vi "Graphical User Interface - Frigg.vi"() -> ()   [LabVIEW 2014]
uses:
  <vilib>/robotics/Controls/Attitude Indicator/Attitude Indicator.xctl
  <vilib>/robotics/Controls/Compass Indicator/Compass Indicator.xctl
  <vilib>/Platform/TimedLoop/XDataNode/timing_clust.ctl
  <vilib>/Platform/TimedLoop/XDataNode/nitl_modes.ctl
  <vilib>/Platform/TimedLoop/XDataNode/wakeup.ctl
  <vilib>/imath/engines/lvmath2/RunTimeEngine/Managers/WorkSpace/UID Generator.vi
  <vilib>/imath/engines/lvmath2/RunTimeEngine/IndexRead/NIMS V(S).vi
  <instcachedir>/0/NIMS V(S)_0488751826AF41519A22953C041130DC.lvgen/NIMS V(S)_0488751826AF41519A22953C041130DC_000.vi
  <vilib>/imath/engines/lvmath2/RunTimeEngine/RunTimeType/NIMS_RunTimeType_From StrictType (excl LVString).vi
  <instcachedir>/0/NIMS_RunTimeType_From StrictType (excl LVString)_15A5391EEA9C4AACB9955AC755B83D29.lvgen/NIMS_RunTimeType_From StrictType (excl LVString)_15A5391EEA9C4AACB9955AC755B83D29_000.vi
  <vilib>/imath/engines/lvmath2/RunTimeEngine/ErrorHandling/NIMS_Create Error From Enums.vi
  <vilib>/imath/engines/lvmath2/RunTimeEngine/LocalVariableDefStatement/MC_LocalVariableDefStatement_Display.vi
  <vilib>/imath/engines/lvmath2/RunTimeEngine/Managers/SymbolTable/Clear UID.vi
  <vilib>/imath/engines/lvmath2/RunTimeEngine/NodeEndStatement/NIMS_NodeEndStatement_Output.vi
  <instcachedir>/0/NIMS_NodeEndStatement_Output_53EC0D466D134D7ABD903AC30B43404B.lvgen/NIMS_NodeEndStatement_Output_53EC0D466D134D7ABD903AC30B43404B_010.vi
  <instcachedir>/0/NIMS_NodeEndStatement_Output_53EC0D466D134D7ABD903AC30B43404B.lvgen/NIMS_NodeEndStatement_Output_53EC0D466D134D7ABD903AC30B43404B_012.vi
  <vilib>/imath/engines/lvmath2/RunTimeEngine/ErrorHandling/NIMS_Finalize Error.vi
  <vilib>/Platform/TimedLoop/XDataNode/XDataNode.xnode
  <vilib>/Platform/TimedLoop/XDataNode/XDNodeRunTimeDep.lvlib
  <vilib>/imath/engines/lvmath2/RunTimeEngine/Managers/SymbolTable/NIMS_WorkSpace.lvlib
panel:
  out "INTERFACE RUNNING":bool
  out "!":bool
  out "Des Head. [deg] 2":dbl format="%#.1f"
  in  "Start New LogFile":bool
  out "Altitide [m]":dbl format="%#.2f"
  out "Des. Altitude":dbl format="%#.2f"
  out "Head. [deg]":dbl format="%#.1f"
  out "Des Head. [deg]":dbl format="%#.1f"
  out "Depth [m]":dbl format="%#.2f"
  out "Des Depth [m]":dbl format="%#.2f"
  out "ALTITUDE":cluster{dbl, dbl}(slide) scale=0.0..10.0
  out "DEPTH":cluster{dbl, dbl}(slide)
  out "DESIRED (red) / ESTIMATED (blue) HEADING":cluster{dbl, dbl}(slide) scale=0.0..360.0
  out "Compass Indicator":dbl(xcontrol)
  out "Attitude Indicator":cluster{"Roll":dbl, "Pitch":dbl}(xcontrol)
  out "POSITION":bool
  in  "Set altitude":bool
  in  "Altitude Button":bool
  in  "Reset Signal \nProcessing":bool
  in  "COLLECTION\nUNIT":bool
  out "Between Setpoints":bool
  out "Auto Par. on Reference Model":bool
  out "MapViewAct":bool
  in  "Reset ROV":bool
  in  "Reset Controller":bool
  in  "Reset Observer":bool
  out "DEPTH":bool
  out "HEADING":bool
  in  "Reset Plots":bool
  in  "Start Button":bool
  out "Using Observer":bool
  in  "SetOrigin":bool
  out "AdvViewAct":bool
  out "ALTITUDE BEAMS":bool[](array[boolean])
  out "Help Field":string
  in  "Vessel Data":bool
  in  "CAMERAS":bool
  in  "MANIPULATOR":bool
  in  "LIGHTS":bool
  out "Status Messages":string[][](table)
  in  "Connect Button":bool
  in  "DP Button":bool
  in  "Stop Button":bool
  in  "Joystick Button":bool
  in  "Tracking Button":bool
  out "SONAR ALT":bool
  out "YAW RATE":bool
  out "SWAY":bool
  out "SURGE":bool
  out "HEADING":bool
  out "DEPTH":bool
  out "EAST":bool
  out "NORTH":bool
  in  "WindowsMediaPlayer":refnum<k7>(container)
  # "AUR-Lab Underwater Operations Control"
  # "ROV info"
  # "SENSORS STATE"
  # "N"
  # "E"
  # "S"
  # "W"
  # "N"
  # "MISSION CONTROL"
  # "DISTANCE ROV-SHIP\non x-y plane"
  # "AUTOPILOT FUNCTIONS"
  # "CONTROL PANEL"
  # "RESET PANEL"
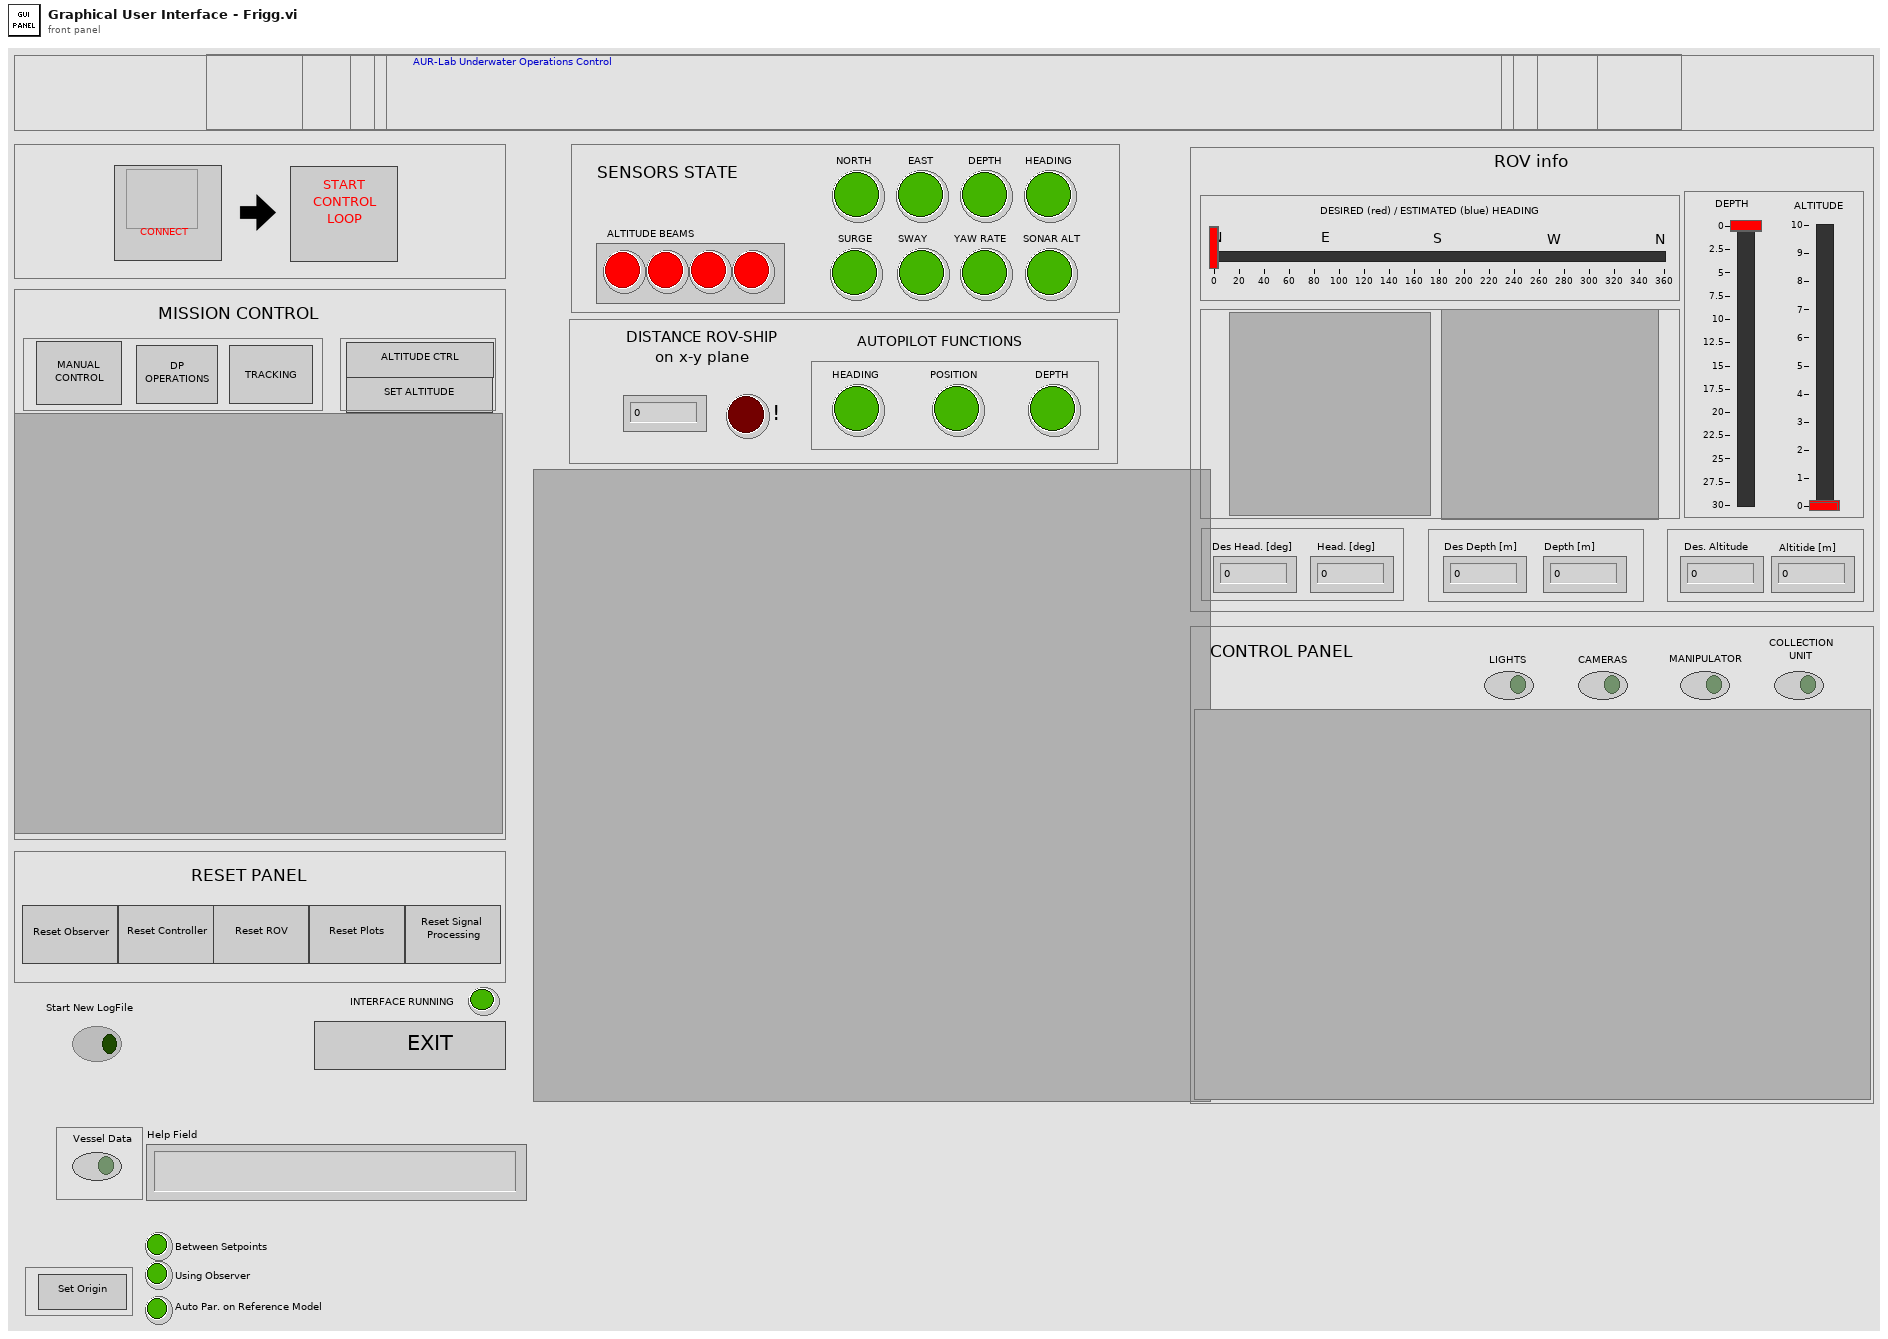
[diagram p1: front panel]
types:
  T1 = enum16{"open", "replace", "create", "open or create", "replace or create", "replace or create with confirmation"}
  T2 = typedef "XDNodeRunTimeDep.lvlib/timing_clust.ctl" = cluster{"Expected End [f-1]":u64, "Actual End [f-1]":u64, "Finished Late? [f-1]":bool, "Expected End [i-1]":u64, "Actual End [i-1]":u64, "Finished Late? [i-1]":bool, "Expected Start [i]":u64, "Actual Start [i]":u64, "Expected Start [f]":u64, "Actual Start [f]":u64, "Source Name":string, "Structure Name":string, "Period":i64, "Deadline":i64, "Offset":i64, "Start":i64, "Priority":i32, "Timeout":i32, "Mode":T3, "Wakeup Reason":T4, "Error":errorcluster, "Source Type":string, "Secondary Source Type":string, "Global End Time":u64, "Global Start Time":u64, "Frame Duration":u64, "Iteration Duration":u64, "Assigned CPU":i32, "I/O Scan Engine Mode":u32}
  T3 = typedef "XDNodeRunTimeDep.lvlib/nitl_modes.ctl" = enum32{"No Change", "Process missed periods, maintain original phase", "Discard missed periods, maintain original phase", "Process missed periods, ignore original phase", "Discard missed periods, ignore original phase"}
  T4 = typedef "XDNodeRunTimeDep.lvlib/wakeup.ctl" = enum32{"Normal", "Aborted", "Asynchronous wakeup", "Timing source error", "Timed loop error", "Timeout"}
  T5 = enum8{"Enabled", "Disabled", "Disabled and Grayed Out"}
  T6 = cluster{"Des Heading [deg]":dbl, "Heading [deg]":dbl}
  T7 = cluster{"Altitude Desired":dbl, "Altitide Estimated":dbl}
  T8 = cluster{"Des Heading [deg]":dbl, "Des Heading [deg]":dbl}
  T9 = cluster{"Shift":bool, "Ctrl":bool, "Alt":bool, "Cmd":bool, "Opt":bool}
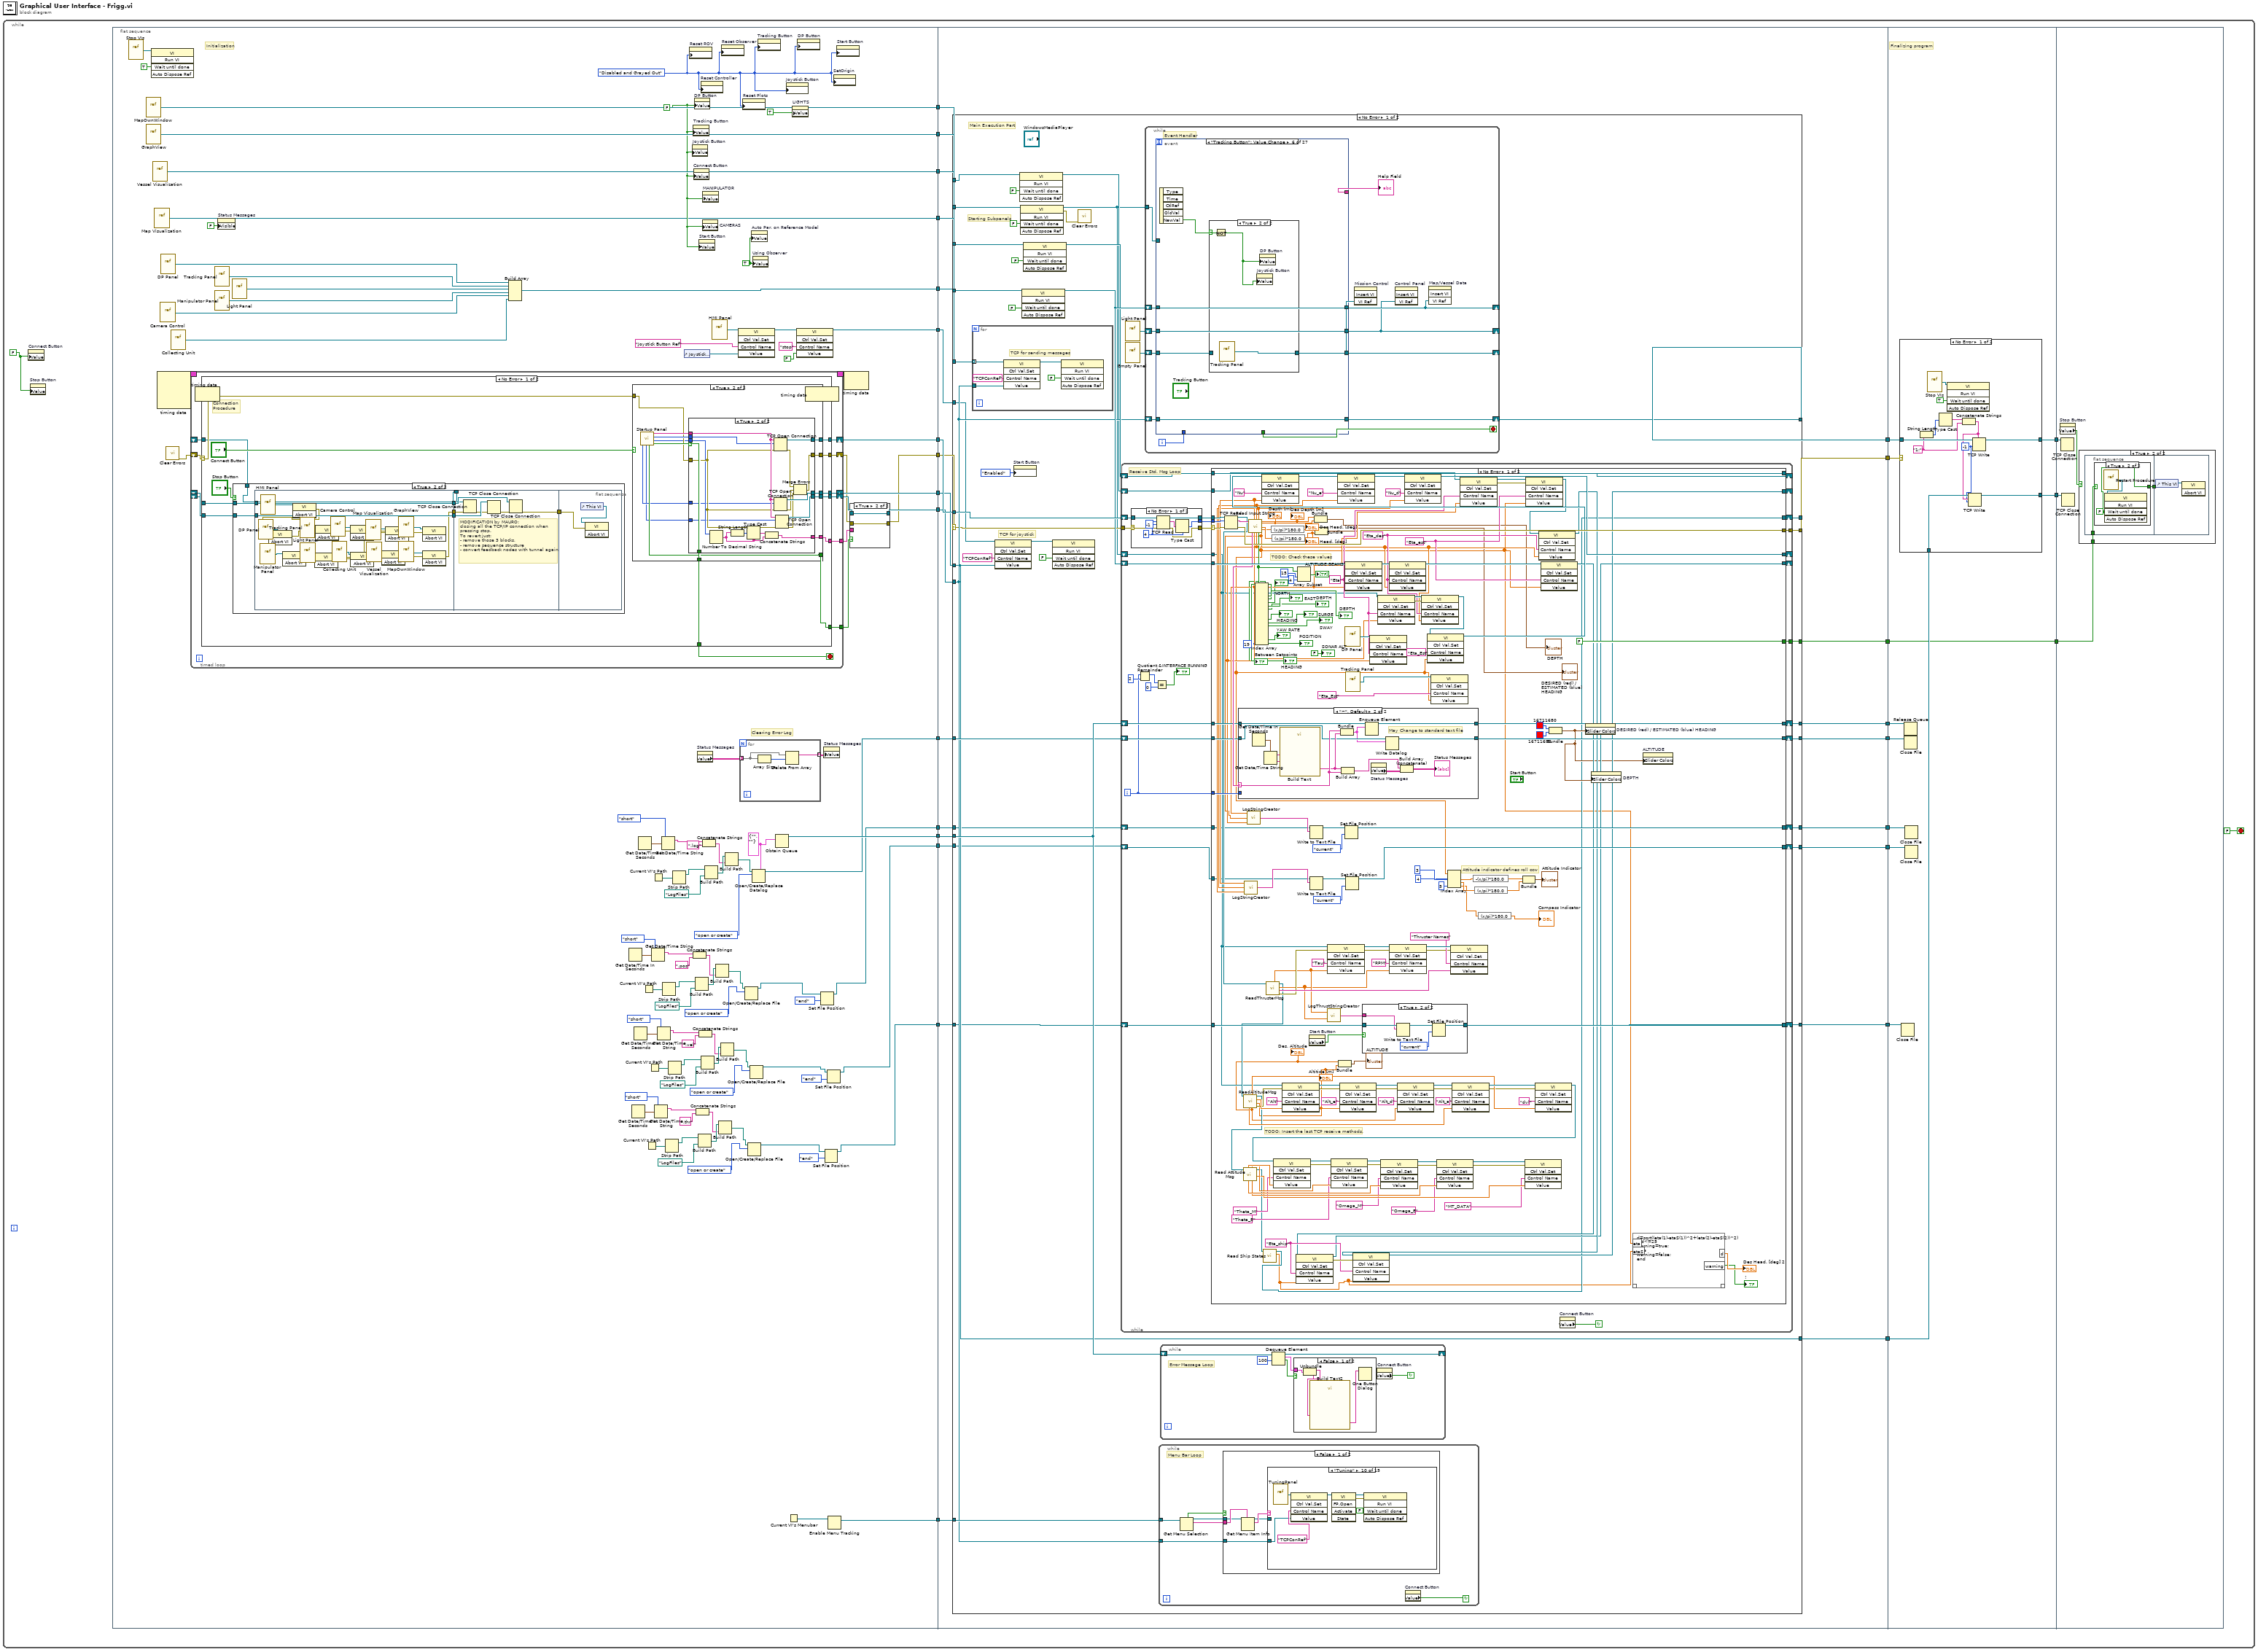
[diagram p0: block diagram]
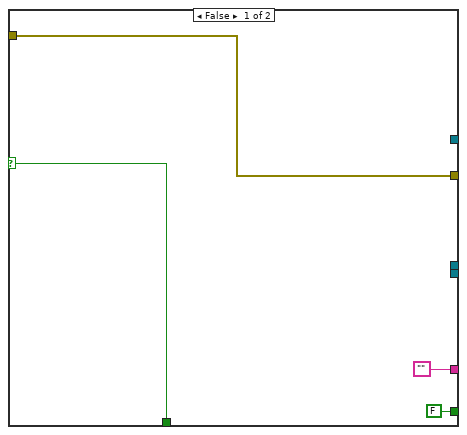
[diagram p3: hidden frame]
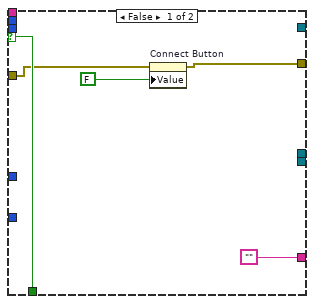
[diagram p4: hidden frame]
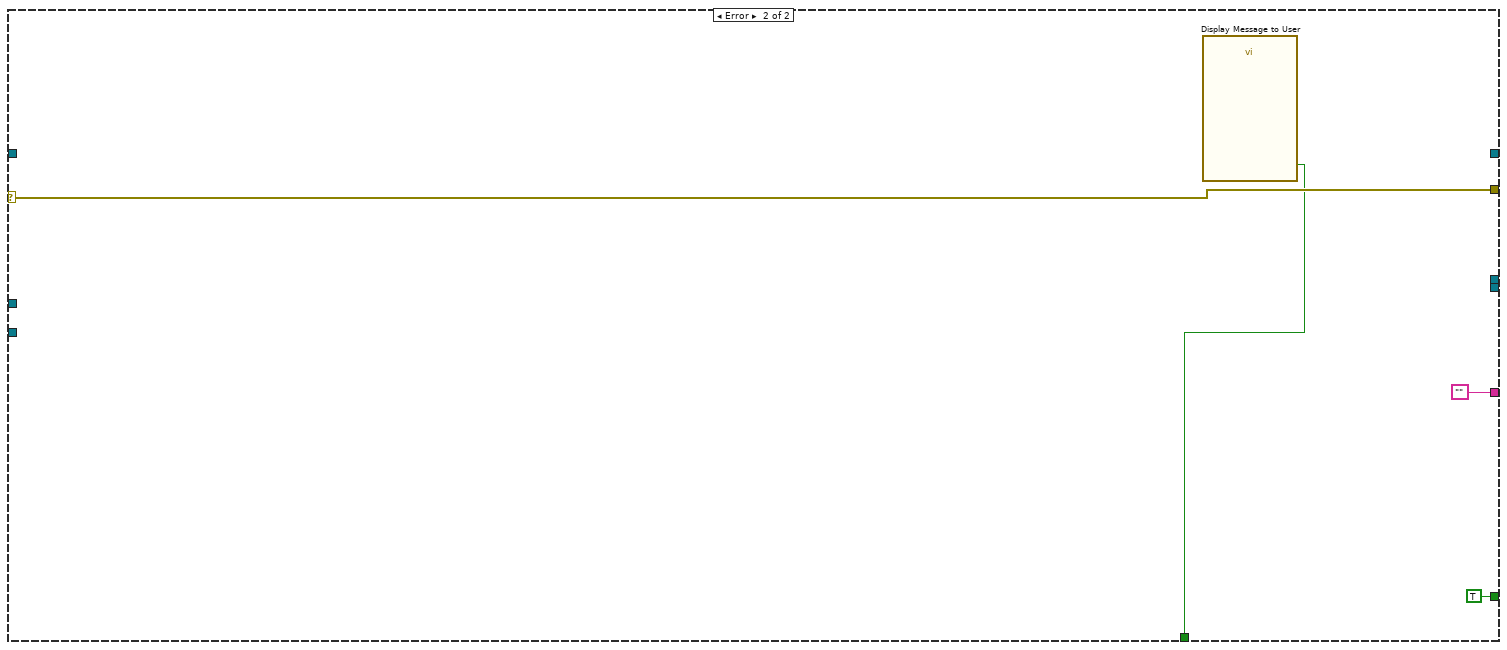
[diagram p5: hidden frame]
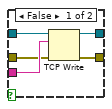
[diagram p6: hidden frame]
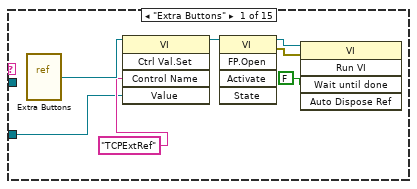
[diagram p7: hidden frame]
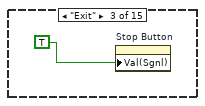
[diagram p9: hidden frame]
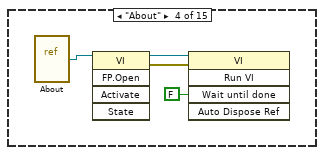
[diagram p10: hidden frame]
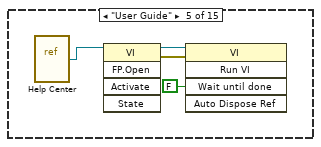
[diagram p11: hidden frame]
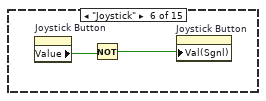
[diagram p12: hidden frame]
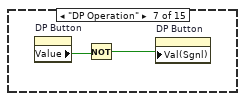
[diagram p13: hidden frame]
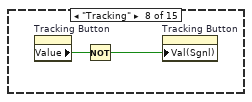
[diagram p14: hidden frame]
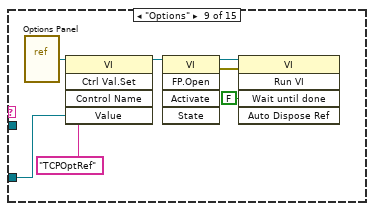
[diagram p15: hidden frame]
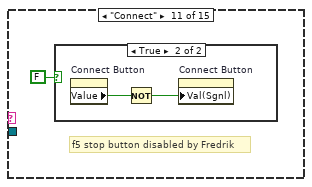
[diagram p16: hidden frame]
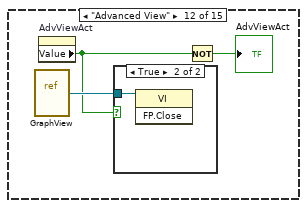
[diagram p18: hidden frame]
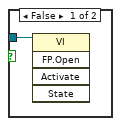
[diagram p19: hidden frame]
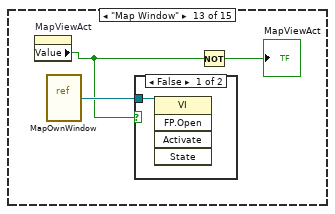
[diagram p20: hidden frame]
diagram:
  n1 = while {
    stop <- FALSE stop-if-true
    w2 = FALSE
    n2 = property on="Connect Button" class="Bool (strict)"("Value"=w2) -> ()  [unwired: 2 in, 2 out]
    n3 = property on="Stop Button" class="Bool (strict)"("Value"=w2) -> ()  [unwired: 2 in, 2 out]
    n4 = flat-sequence {
      tunnel: [w126] -> w30
      tunnel: [w31] -> w29
      tunnel: [w123] -> w28
      tunnel: [w117] -> w27
      tunnel: [w32] -> w26
      tunnel: [w113] -> w25
      tunnel: [w109] -> w23
      tunnel: [w107] -> w19
      tunnel: [w51] -> w18
      tunnel: [w54] -> w14
      tunnel: [w104] -> w13
      tunnel: [w91] -> w12
      tunnel: [w40] -> w8
      tunnel: [w38] -> w6
      tunnel: [w36] -> w5
      tunnel: [w57] -> w3
      tunnel: w30 -> [w271]
      tunnel: [w251] -> w22
      tunnel: w29 -> [w274]
      tunnel: w28 -> [w273]
      tunnel: w27 -> [w272]
      tunnel: w26 -> [w270]
      tunnel: w25 -> [w269]
      tunnel: [w264] -> w21
      tunnel: w23 -> [w268]
      tunnel: [w267] -> w20
      tunnel: w19 -> [w266]
      tunnel: w18 -> [w265]
      tunnel: [w263] -> w17
      tunnel: [w262] -> w15
      tunnel: w14 -> [w261]
      tunnel: w13 -> [w260]
      tunnel: w12 -> [w259]
      tunnel: [w258] -> w11
      tunnel: w8 -> [w257]
      tunnel: [w256] -> w7
      tunnel: w6 -> [w254]
      tunnel: w5 -> [w255]
      tunnel: [w253] -> w4
      tunnel: w3 -> [w252]
      tunnel: [w250] -> w1
      tunnel: w22 -> [w1109]
      tunnel: w21 -> [w1108]
      tunnel: w20 -> [w1107]
      tunnel: w17 -> [w1106]
      tunnel: [w1105] -> w16
      tunnel: w15 -> [w1105]
      tunnel: w11 -> [w1104]
      tunnel: [w1103] -> w10
      tunnel: [w1102] -> w9
      tunnel: w7 -> [w1101]
      tunnel: w4 -> [w1100]
      tunnel: w1 -> [w1099]
      tunnel: w16 -> [w1128]
      tunnel: w10 -> [w1127]
      tunnel: w9 -> [w1126]
      frame #0 {
        w50 = T5."Disabled and Grayed Out" ("Disabled")
        w56 = TRUE ("Using Observer")
        w92 = cluster{string, string} {"", ""}
        w43 = FALSE
        # "Clearing Error Log"
        # "Initialization"
        n5 = vi-ref "Stop VIs.vi"() -> (w48:refnum<vi>)
        n6 = vi-ref "MapOwnWindow.vi"() -> (w57:refnum<vi>)
        n7 = vi-ref "GraphView.vi"() -> (w104:refnum<vi>)
        n8 = invoke class="VI" method="Run VI"(reference=w48, "Wait until done"=TRUE ("Wait Until Done")) -> ()  [unwired: 3 in, 5 out]
        n9 = vi-ref "Vessel Visualization.vi"() -> (w123:refnum<vi>)
        n10 = vi-ref "Map Visualization.vi"() -> (w31:refnum<vi>)
        n11 = node-c288() -> (w46:T2)  [unwired: 4 in]
        n12 = vi-ref "Camera Control.vi"() -> (w118:refnum<vi>)
        n13 = vi-ref "DP Panel.vi"() -> (w122:refnum<vi>)
        n14 = call <vilib>:"Clear Errors.vi"() -> ("error out"=w105:errorcluster)  [unwired: 6 in, 1 out]
        n15 = vi-ref "Collecting Unit.vi"() -> (w44:refnum<vi>)
        n16 = timed-loop {
          shift-right: [w134] -> w52
          shift-left: w105 -> [w133]
          tunnel: [w131] -> w55
          tunnel: [w130] -> w47
          timing: w46 -> [_]
          timing-out: [_] -> w45
          shift-right: [w137] -> w126
          shift-left: _ -> [w129]
          shift-right: [w136] -> w113
          shift-left: _ -> [w128]
          shift-right: [w132] -> w53
          shift-left: _ -> [w127]
          stop <- w135 stop-if-true
          n17 = node-c288() -> ()  [unwired: 1 in, 1 out]
          n18 = case shown="No Error" w133 {
            selector: w133 -> [w147 w237]
            tunnel: [w152 _] -> w137
            tunnel: [w151 _] -> w136
            tunnel: [w150 w236] -> w135
            tunnel: [w148 w237] -> w134
            tunnel: [w146 _] -> w132
            tunnel: [w145 ""] -> w131
            tunnel: [w143 TRUE ("Restart Out")] -> w130
            tunnel: w129 -> [w140 _]
            tunnel: w128 -> [w142 _]
            tunnel: w127 -> [w141 _]
            frame No Error {
              # "Connection\nProcedure"
              n19 = case shown="True" "Stop Button" {
                tunnel: w142 -> [_ w159]
                tunnel: w141 -> [_ w158]
                tunnel: w140 -> [_ w155]
                frame False {
                }
                frame True {
                  n20 = flat-sequence {
                    tunnel: w158 -> [w182]
                    tunnel: w159 -> [w183]
                    tunnel: [w183] -> w157
                    tunnel: [w182] -> w156
                    tunnel: [w160] -> w154
                    tunnel: w157 -> [w190]
                    tunnel: w156 -> [w189]
                    tunnel: w155 -> [w188]
                    tunnel: w154 -> [w187]
                    tunnel: [w184] -> w153
                    tunnel: w153 -> [w191]
                    frame #0 {
                      n21 = vi-ref "DP Panel.vi"() -> (w181:refnum<vi>)
                      n22 = vi-ref "Manipulator Panel.vi"() -> (w176:refnum<vi>)
                      n23 = vi-ref "HMI Panel.vi"() -> (w162:refnum<vi>)
                      n24 = invoke class="VI" method="Abort VI"(reference=w162) -> (error out=w161:errorcluster)  [unwired: 2 in, 2 out]
                      n25 = invoke class="VI" method="Abort VI"(reference=w181, error in=w161) -> (error out=w171:errorcluster)  [unwired: 1 in, 2 out]
                      n26 = vi-ref "Tracking Panel.vi"() -> (w180:refnum<vi>)
                      n27 = vi-ref "Light Panel.vi"() -> (w175:refnum<vi>)
                      n28 = invoke class="VI" method="Abort VI"(reference=w180, error in=w171) -> (error out=w170:errorcluster)  [unwired: 1 in, 2 out]
                      n29 = vi-ref "Camera Control.vi"() -> (w179:refnum<vi>)
                      n30 = vi-ref "Collecting Unit.vi"() -> (w174:refnum<vi>)
                      n31 = invoke class="VI" method="Abort VI"(reference=w179, error in=w170) -> (error out=w169:errorcluster)  [unwired: 1 in, 2 out]
                      n32 = vi-ref "Map Visualization.vi"() -> (w178:refnum<vi>)
                      n33 = vi-ref "Vessel Visualization.vi"() -> (w173:refnum<vi>)
                      n34 = invoke class="VI" method="Abort VI"(reference=w178, error in=w169) -> (error out=w168:errorcluster)  [unwired: 1 in, 2 out]
                      n35 = vi-ref "GraphView.vi"() -> (w177:refnum<vi>)
                      n36 = vi-ref "MapOwnWindow.vi"() -> (w172:refnum<vi>)
                      n37 = invoke class="VI" method="Abort VI"(reference=w177, error in=w168) -> (error out=w167:errorcluster)  [unwired: 1 in, 2 out]
                      n38 = invoke class="VI" method="Abort VI"(reference=w176, error in=w167) -> (error out=w166:errorcluster)  [unwired: 1 in, 2 out]
                      n39 = invoke class="VI" method="Abort VI"(reference=w175, error in=w166) -> (error out=w165:errorcluster)  [unwired: 1 in, 2 out]
                      n40 = invoke class="VI" method="Abort VI"(reference=w174, error in=w165) -> (error out=w164:errorcluster)  [unwired: 1 in, 2 out]
                      n41 = invoke class="VI" method="Abort VI"(reference=w173, error in=w164) -> (error out=w163:errorcluster)  [unwired: 1 in, 2 out]
                      n42 = invoke class="VI" method="Abort VI"(reference=w172, error in=w163) -> (error out=w160:errorcluster)  [unwired: 1 in, 2 out]
                    }
                    frame #1 {
                      # "MODIFICATION by MAURO:\nclosing all the TCP/IP connection when\npressing stop.\nTo revert just:\n- remove those 3 blocks, \n- remove sequence structure\n- convert feedback nodes with tunnel again"
                      n43 = TCP Close Connection(connection ID=w188, error in (no error)=w187) -> (error out=w186:errorcluster)  [unwired: 1 in, 1 out]
                      n44 = TCP Close Connection(connection ID=w190, error in (no error)=w186) -> (error out=w185:errorcluster)  [unwired: 1 in, 1 out]
                      n45 = TCP Close Connection(connection ID=w189, error in (no error)=w185) -> (error out=w184:errorcluster)  [unwired: 1 in, 1 out]
                    }
                    frame #2 {
                      n46 = control-ref of="This VI"() -> (w192:refnum<vi>)
                      n47 = invoke class="VI" method="Abort VI"(reference=w192, error in=w191) -> ()  [unwired: 1 in, 3 out]
                    }
                  }
                }
              }
              n48 = case shown="True" "Connect Button" {
                selector: "Connect Button" -> [w196 _]
                tunnel: [_ w210] -> w152
                tunnel: [_ w209] -> w151
                tunnel: [w196 w208] -> w150
                tunnel: [w195 w207] -> w148
                tunnel: w147 -> [w195 w202]
                tunnel: [_ w206] -> w146
                tunnel: ["" w200] -> w145
                tunnel: [FALSE ("Restart Out") w199] -> w143
                frame False {
                }
                frame True {
                  n49 = call "Startup Panel.vi"() -> ("Bool Out"=w204:bool, "ROV Selector Out"=w201:u16, "Port Number Recv Out 1"=w203:u16, "IP Address Out"=w205:string, "Restart Out"=w199:bool, "Port Number  Send Out"=w197:u16, "Port Number Joyst. Out"=w198:u16)  [unwired: 5 in]
                  n50 = case shown="True" w204 {
                    selector: w204 -> [w214 w230]
                    tunnel: [_ w233] -> w210
                    tunnel: [_ w232] -> w209
                    tunnel: w205 -> [_ w231]
                    tunnel: w203 -> [_ w224]
                    tunnel: [w214 w230] -> w208
                    tunnel: w202 -> [w213 w228]
                    tunnel: [w212 w225] -> w207
                    tunnel: [_ w229] -> w206
                    tunnel: w201 -> [_ w223]
                    tunnel: ["" w219] -> w200
                    tunnel: w198 -> [_ w218]
                    tunnel: w197 -> [_ w217]
                    frame False {
                      n51 = property on="Connect Button" class="Bool (strict)"(error in=w213, "Value"=FALSE ("Connect Button")) -> (error out=w212:errorcluster)  [unwired: 1 in, 1 out]
                    }
                    frame True {
                      n52 = Number To Decimal String(number=w223) -> (decimal integer string=w220:string)  [unwired: 1 in]
                      n53 = String Length(string=w220) -> (length=w222:i32)
                      n54 = Type Cast(type=w220, x=w222) -> (*(type *) &x=w221:string)
                      n55 = Concatenate Strings(w221, w220) -> (w219:string)
                      n56 = TCP Open Connection(address=w231, remote port or service name=w224, error in (no error)=w228) -> (connection ID=w233:refnum<k5>, error out=w216:errorcluster)  [unwired: 2 in]
                      n57 = TCP Open Connection(address=w231, remote port or service name=w218, error in (no error)=w228) -> (connection ID=w232:refnum<k5>, error out=w227:errorcluster)  [unwired: 2 in]
                      n58 = TCP Open Connection(address=w231, remote port or service name=w217, error in (no error)=w228) -> (connection ID=w229:refnum<k5>, error out=w226:errorcluster)  [unwired: 2 in]
                      n59 = Merge Errors(w216, w227, w226) -> (w225:errorcluster)
                    }
                  }
                }
              }
            }
            frame Error {
              n60 = call "Display Message to User"() -> ("OK"=w236:bool)  [unwired: 10 in, 1 out]
            }
          }
          n61 = node-c288() -> ()  [unwired: 1 in, 1 out]
        }
        n62 = vi-ref "Tracking Panel.vi"() -> (w121:refnum<vi>)
        n63 = vi-ref "Manipulator Panel.vi"() -> (w119:refnum<vi>)
        n64 = property on="Status Messages" class="Tbl (strict)"("Visible"=FALSE) -> ()  [unwired: 2 in, 2 out]
        n65 = vi-ref "Light Panel.vi"() -> (w120:refnum<vi>)
        n66 = Build Array(w122, w121, w120, w119, w118, w44) -> (w117:refnum<vi>[])
        n67 = Get Date/Time In Seconds() -> (seconds since 1Jan1904=w87:timestamp)
        n68 = Get Date/Time In Seconds() -> (seconds since 1Jan1904=w65:timestamp)
        n69 = Get Date/Time In Seconds() -> (seconds since 1Jan1904=w76:timestamp)
        n70 = Get Date/Time In Seconds() -> (seconds since 1Jan1904=w100:timestamp)
        n71 = Current VI's Path() -> (path=w90:path)
        n72 = Current VI's Path() -> (path=w68:path)
        n73 = Current VI's Path() -> (path=w79:path)
        n74 = Get Date/Time String(date format (0)=enum16{"short", "long", "abbreviated"}."short", seconds (now)=w87) -> (date string=w86:string)  [unwired: 1 in, 1 out]
        n75 = Current VI's Path() -> (path=w103:path)
        n76 = Get Date/Time String(date format (0)=enum16{"short", "long", "abbreviated"}."short", seconds (now)=w65) -> (date string=w64:string)  [unwired: 1 in, 1 out]
        n77 = Get Date/Time String(date format (0)=enum16{"short", "long", "abbreviated"}."short", seconds (now)=w76) -> (date string=w75:string)  [unwired: 1 in, 1 out]
        n78 = Get Date/Time String(date format (0)=enum16{"short", "long", "abbreviated"}."short", seconds (now)=w100) -> (date string=w99:string)  [unwired: 1 in, 1 out]
        n79 = Strip Path(path=w90) -> (stripped path=w89:path)  [unwired: 1 out]
        n80 = Strip Path(path=w68) -> (stripped path=w67:path)  [unwired: 1 out]
        n81 = Strip Path(path=w79) -> (stripped path=w78:path)  [unwired: 1 out]
        n82 = Strip Path(path=w103) -> (stripped path=w102:path)  [unwired: 1 out]
        n83 = control-ref of="Joystick Button"() -> (w115:refnum<vi>)
        n84 = property on="Reset ROV" class="Bool"("DisabledEnum"=w50) -> ()  [unwired: 2 in, 2 out]
        n85 = property on="Joystick Button" class="Bool (strict)"("Value"=w43) -> ()  [unwired: 2 in, 2 out]
        n86 = property on="Tracking Button" class="Bool (strict)"("Value"=w43) -> ()  [unwired: 2 in, 2 out]
        n87 = Concatenate Strings(w86, ".pos" ("string")) -> (w83:string)
        n88 = property on="Connect Button" class="Bool (strict)"("Value"=w43) -> ()  [unwired: 2 in, 2 out]
        n89 = property on="DP Button" class="Bool (strict)"("Value"=w43) -> ()  [unwired: 2 in, 2 out]
        n90 = Build Path(base path=w89, name or relative path=path "LogFiles") -> (appended path=w84:path)
        n91 = Concatenate Strings(w64, ".thr" ("string")) -> (w61:string)
        n92 = property on="Status Messages" class="Tbl (strict)"() -> ("Value"=w125:string[][])  [unwired: 2 in, 2 out]
        n93 = Build Path(base path=w67, name or relative path=path "LogFiles") -> (appended path=w62:path)
        n94 = Concatenate Strings(w75, ".vel" ("string")) -> (w72:string)
        n95 = property on="Start Button" class="Bool (strict)"("Value"=w43) -> ()  [unwired: 2 in, 2 out]
        n96 = property on="Reset Controller" class="Bool"("DisabledEnum"=w50) -> ()  [unwired: 2 in, 2 out]
        n97 = Build Path(base path=w78, name or relative path=path "LogFiles") -> (appended path=w73:path)
        n98 = property on="CAMERAS" class="Bool (strict)"("Value"=w43) -> ()  [unwired: 2 in, 2 out]
        n99 = property on="MANIPULATOR" class="Bool (strict)"("Value"=w43) -> ()  [unwired: 2 in, 2 out]
        n100 = Concatenate Strings(w99, ".log" ("string")) -> (w96:string)
        n101 = Build Path(base path=w102, name or relative path=path "LogFiles") -> (appended path=w97:path)
        n102 = vi-ref "HMI Panel.vi"() -> (w116:refnum<vi>)
        n103 = Build Path(base path=w84, name or relative path=w83) -> (appended path=w81:path)
        n104 = Build Path(base path=w62, name or relative path=w61) -> (appended path=w60:path)
        n105 = Build Path(base path=w73, name or relative path=w72) -> (appended path=w71:path)
        n106 = property on="Reset Observer" class="Bool"("DisabledEnum"=w50) -> ()  [unwired: 2 in, 2 out]
        n107 = Build Path(base path=w97, name or relative path=w96) -> (appended path=w93:path)
        n108 = invoke class="VI" method="Ctrl Val.Set"(reference=w116, "Control Name"="Joystick Button Ref", "Value"=w115) -> (reference out=w110:refnum<vi>)  [unwired: 2 in, 4 out]
        n109 = for {
          tunnel: w125 -> [w248] mode=indexing
          tunnel: [w247] -> w124 mode=indexing
          n110 = Array Size(array=w248) -> (size(s)=w249:i32)
          n111 = Delete From Array(array=w248, length=w249) -> (array with subset deleted=w247:string[])  [unwired: 1 in, 1 out]
        }
        n112 = property on="Reset Plots" class="Bool"("DisabledEnum"=w50) -> ()  [unwired: 2 in, 2 out]
        n113 = Open/Create/Replace File(file path (use dialog)=w81, operation (0:open)=T1."open or create") -> (refnum out=w41:refnum<file>)  [unwired: 4 in, 2 out]
        n114 = Open/Create/Replace File(file path (use dialog)=w60, operation (0:open)=T1."open or create") -> (refnum out=w37:refnum<file>)  [unwired: 4 in, 2 out]
        n115 = Open/Create/Replace File(file path (use dialog)=w71, operation (0:open)=T1."open or create") -> (refnum out=w39:refnum<file>)  [unwired: 4 in, 2 out]
        n116 = property on="Auto Par. on Reference Model" class="Bool (strict)"("Value"=w56) -> ()  [unwired: 2 in, 2 out]
        n117 = Open/Create/Replace Datalog(5:w92, 10:T1."open or create" ("operation (0:open)"), 11:w93) -> (3:w91:refnum<k1>)  [unwired: 3 in, 2 out]
        n118 = property on="Using Observer" class="Bool (strict)"("Value"=w56) -> ()  [unwired: 2 in, 2 out]
        n119 = property on="Tracking Button" class="Bool (strict)"("DisabledEnum"=w50) -> ()  [unwired: 2 in, 2 out]
        n120 = Obtain Queue(element data type=w92) -> (queue out=w109:refnum<queue>)  [unwired: 4 in, 2 out]
        n121 = property on="Joystick Button" class="Bool (strict)"("DisabledEnum"=w50) -> ()  [unwired: 2 in, 2 out]
        n122 = Current VI's Menubar() -> (w108:refnum<k9>)
        n123 = property on="LIGHTS" class="Bool (strict)"("Value"=TRUE) -> ()  [unwired: 2 in, 2 out]
        n124 = invoke class="VI" method="Ctrl Val.Set"(reference=w110, "Control Name"="stop", "Value"=FALSE) -> (reference out=w32:refnum<vi>)  [unwired: 2 in, 4 out]
        n125 = property on="DP Button" class="Bool (strict)"("DisabledEnum"=w50) -> ()  [unwired: 2 in, 2 out]
        n126 = Set File Position(refnum=w41, from (0:start)=enum16{"start", "end", "current"}."end") -> (refnum out=w40:refnum<file>)  [unwired: 2 in, 1 out]
        n127 = property on="Status Messages" class="Tbl (strict)"("Value"=w124) -> ()  [unwired: 2 in, 2 out]
        n128 = Set File Position(refnum=w37, from (0:start)=enum16{"start", "end", "current"}."end") -> (refnum out=w36:refnum<file>)  [unwired: 2 in, 1 out]
        n129 = Set File Position(refnum=w39, from (0:start)=enum16{"start", "end", "current"}."end") -> (refnum out=w38:refnum<file>)  [unwired: 2 in, 1 out]
        n130 = Enable Menu Tracking(4:w108) -> (1:w107:refnum<k9>)  [unwired: 2 in, 1 out]
        n131 = property on="SetOrigin" class="Bool"("DisabledEnum"=w50) -> ()  [unwired: 2 in, 2 out]
        n132 = property on="Start Button" class="Bool (strict)"("DisabledEnum"=w50) -> ()  [unwired: 2 in, 2 out]
        n133 = node-c288(w45) -> ()  [unwired: 1 out]
        n134 = case shown="True" w47 {
          tunnel: w55 -> [w244 _]
          tunnel: [w243 w246] -> w54
          tunnel: w53 -> [w242 w246]
          tunnel: w52 -> [w241 w245]
          tunnel: [w240 w245] -> w51
          frame False {
            n135 = TCP Write(connection ID=w242, data in=w244, error in (no error)=w241) -> (connection ID out=w243:refnum<k5>, error out=w240:errorcluster)  [unwired: 1 in, 1 out]
          }
          frame True {
          }
        }
      }
      frame #1 {
        n136 = case shown="No Error" w265 {
          selector: w265 -> [w290 w1092]
          tunnel: [w314 w1097] -> _
          tunnel: w274 -> [w310 _]
          tunnel: w273 -> [w309 _]
          tunnel: w272 -> [w308 _]
          tunnel: w271 -> [w307 w1097]
          tunnel: w270 -> [w275 _]
          tunnel: w269 -> [w289 w1096]
          tunnel: w268 -> [w300 w1098]
          tunnel: [w299 w1098] -> w267
          tunnel: w266 -> [w298 _]
          tunnel: [w289 w1096] -> w264
          tunnel: [w297 w1092] -> w263
          tunnel: [w296 w1090] -> w262
          tunnel: w261 -> [w291 w1085]
          tunnel: w260 -> [w295 _]
          tunnel: w259 -> [w293 w1089]
          tunnel: [w292 w1089] -> w258
          tunnel: w257 -> [w288 w1088]
          tunnel: [w287 w1088] -> w256
          tunnel: w255 -> [w279 w1086]
          tunnel: w254 -> [w286 w1087]
          tunnel: [w285 w1087] -> w253
          tunnel: w252 -> [w284 _]
          tunnel: [w280 w1085] -> w251
          tunnel: [w278 w1086] -> w250
          frame No Error {
            # "TCP for joystick"
            # "Starting Subpanels"
            # "Main Execution Part"
            n137 = for {
              tunnel: w308 -> [w739] mode=indexing
              tunnel: w291 -> [w738]
              # "TCP for sending messages"
              n138 = invoke class="VI" method="Ctrl Val.Set"(reference=w739, "Control Name"="TCPConRef", "Value"=w738) -> (reference out=w741:refnum<vi>)  [unwired: 2 in, 4 out]
              n139 = invoke class="VI" method="Run VI"(reference=w741, "Wait until done"=FALSE) -> ()  [unwired: 3 in, 5 out]
            }
            n140 = invoke class="VI" method="Ctrl Val.Set"(reference=w275, "Control Name"="TCPConRef", "Value"=w289) -> (reference out=w302:refnum<vi>)  [unwired: 2 in, 4 out]
            n141 = property on="Start Button" class="Bool (strict)"("DisabledEnum"=T5."Enabled" ("Disabled")) -> ()  [unwired: 2 in, 2 out]
            n142 = invoke class="VI" method="Run VI"(reference=w284, "Wait until done"=FALSE ("Wait Until Done")) -> (reference out=w282:refnum<vi>)  [unwired: 3 in, 4 out]
            n143 = invoke class="VI" method="Run VI"(reference=w295, "Wait until done"=FALSE ("Wait Until Done")) -> (reference out=w277:refnum<vi>, error out=w276:errorcluster)  [unwired: 3 in, 3 out]
            n144 = invoke class="VI" method="Run VI"(reference=w310, "Wait until done"=FALSE) -> (reference out=w306:refnum<vi>)  [unwired: 3 in, 4 out]
            n145 = invoke class="VI" method="Run VI"(reference=w309, "Wait until done"=FALSE) -> (reference out=w305:refnum<vi>)  [unwired: 3 in, 4 out]
            n146 = invoke class="VI" method="Run VI"(reference=w302, "Wait until done"=FALSE) -> ()  [unwired: 3 in, 5 out]
            n147 = call <vilib>:"Clear Errors.vi"("error in (no error)"=w276) -> ()  [unwired: 5 in, 2 out]
            n148 = while "Timed Loop" {
              shift-right: [w429] -> w314
              shift-left: w307 -> [w432]
              shift-right: [w428] -> _
              shift-left: w306 -> [w406]
              shift-right: [w426] -> _
              shift-left: w305 -> [w427]
              shift-right: [w424] -> w299
              shift-left: w300 -> [w425]
              tunnel: w290 -> [w423]
              tunnel: [w420] -> w297
              tunnel: [w419] -> w296
              shift-right: [w417] -> _
              shift-left: w277 -> [w418]
              shift-right: [w416] -> w292
              shift-left: w293 -> [w415]
              shift-right: [w413] -> w287
              shift-left: w288 -> [w414]
              shift-right: [w411] -> w285
              shift-left: w286 -> [w412]
              shift-right: [w410] -> _
              shift-left: w282 -> [w407]
              shift-right: [w409] -> w278
              shift-left: w279 -> [w408]
              i -> [w402]
              stop <- w421 continue-if-true
              # "Receive Std. Msg Loop"
              n149 = case shown="No Error" w423 {
                selector: w423 -> [w729 w737]
                tunnel: w432 -> [w734 w736]
                tunnel: [w733 w736] -> w431
                tunnel: [w730 0] -> w430
                tunnel: [w728 w737] -> w422
                frame No Error {
                  w731 = 4
                  n150 = TCP Read(connection ID=w734, bytes to read=w731, error in (no error)=w729, 9:-1 ("timeout ms (25000)")) -> (connection ID out=w733:refnum<k5>, data out=w732:string, error out=w728:errorcluster)  [unwired: 1 in]
                  n151 = Type Cast(type=w731, x=w732) -> (*(type *) &x=w730:i32)
                }
                frame Error {
                }
              }
              n152 = Quotient & Remainder(x=w402, y=2) -> (x-y*floor(x/y)=w401:i32)  [unwired: 1 out]
              n153 = Equal?(x=w401, y=0) -> (x = y?=→"INTERFACE RUNNING":bool)
              n154 = case shown="No Error" w422 {
                selector: w422 -> [w577 w721]
                tunnel: w431 -> [w591 w723]
                tunnel: w430 -> [w590 _]
                tunnel: [w439 w723] -> w429
                tunnel: w406 -> [w589 w725]
                tunnel: [w470 w725] -> w428
                tunnel: w427 -> [w558 w726]
                tunnel: [w558 w726] -> w426
                tunnel: w402 -> [w582 _]
                tunnel: w425 -> [w581 w724]
                tunnel: [w580 w724] -> w424
                tunnel: [w576 w721] -> w420
                tunnel: [FALSE ("Yes") w717] -> w419
                tunnel: w418 -> [w503 w716]
                tunnel: [w559 w716] -> w417
                tunnel: [w566 w715] -> w416
                tunnel: w415 -> [w565 w715]
                tunnel: w414 -> [w478 w714]
                tunnel: [w557 w714] -> w413
                tunnel: w412 -> [w477 w713]
                tunnel: [w552 w713] -> w411
                tunnel: w407 -> [w547 w712]
                tunnel: [w473 w712] -> w410
                tunnel: [w524 w711] -> w409
                tunnel: w408 -> [w523 w711]
                frame No Error {
                  w474 = "Eta_ship" ("Control Name")
                  w542 = "Eta_est" ("Control Name")
                  w540 = "Eta_des"
                  w546 = "Eta"
                  # "Attitude indicator defines roll ccw"
                  # "TODO: Insert the last TCP receive methods."
                  # "TODO: Check these values"
                  n155 = TCP Read(connection ID=w591, bytes to read=w590, error in (no error)=w577) -> (connection ID out=w505:refnum<k5>, data out=w592:string, error out=w576:errorcluster)  [unwired: 2 in]
                  n156 = call "Read Input String.vi"("Input"=w592) -> ("Msg Out"=w587:string, "Nu"=w555:dbl[], "Eta"=w545:dbl[], "Nu_est"=w554:dbl[], "Eta_d"=w539:dbl[], "Nu_d"=w548:dbl[], "Array"=w573:bool[], "Des Depth [m]"=w449:dbl, "Depth [m]"=w448:dbl, "Heading [deg]"=w579:dbl, "Des Heading [deg]"=w564:dbl, "Eta_est"=w433:dbl[])  [unwired: 7 in]
                  "Des Depth [m]" <- w449
                  "Depth [m]" <- w448
                  n157 = case shown="\"~\", Default" w587 {
                    selector: w587 -> [_ w702]
                    tunnel: w582 -> [_ _]
                    tunnel: w581 -> [w697 w704]
                    tunnel: [w697 w703] -> w580
                    tunnel: [w696 w699] -> w566
                    tunnel: w565 -> [w696 w700]
                    frame "OK" {
                    }
                    frame "~", Default {
                      # "May Change to standard text file"
                      n158 = Get Date/Time In Seconds() -> (seconds since 1Jan1904=w710:timestamp)
                      n159 = Get Date/Time String(seconds (now)=w710) -> (date string=w709:string, time string=w708:string)  [unwired: 2 in]
                      n160 = call "Build Text"("Date"=w709, "Time"=w708) -> ("Result"=w701:string)  [unwired: 12 in, 1 out]
                      n161 = Bundle(w702, "Result"=w701) -> (w698:cluster{string, "Result":string})  [unwired: 1 in]
                      n162 = Build Array(w701, w702) -> (w706:string[])
                      n163 = Enqueue Element(queue=w704, element=w698) -> (queue out=w703:refnum<queue>)  [unwired: 2 in, 2 out]
                      n164 = property on="Status Messages" class="Tbl (strict)"() -> ("Value"=w707:string[][])  [unwired: 2 in, 2 out]
                      n165 = Write Datalog(6:w698, 7:w700) -> (3:w699:refnum<k1>)  [unwired: 1 in, 1 out]
                      n166 = Build Array (concatenate)(w706, w707) -> (→"Status Messages":string[][])
                    }
                  }
                  n167 = call "LogStringCreator.vi"("Eta_d"=w548, "Eta_e"=w554, "Eta"=w555) -> ("Output"=w553:string)
                  n168 = call "LogStringCreator.vi"("Eta_d"=w539, "Eta_e"=w433, "Eta"=w545) -> ("Output"=w556:string)
                  n169 = Index Array(array=w573, index #16=19 ("index")) -> (element #1=→"Between Setpoints":bool, element #2=→"DEPTH":bool, element #3=→"HEADING":bool, element #4=→"NORTH":bool, element #5=→"EAST":bool, element #6=→"DEPTH":bool, element #9=→"HEADING":bool, element #10=→"SURGE":bool, element #11=→"SWAY":bool, element #15=→"YAW RATE":bool, element #16=→"POSITION":bool)  [unwired: 15 in, 5 out]
                  n170 = call "ReadThrusterMsg.vi"("TCPCon In"=w505) -> ("Error Out"=w531:errorcluster, "Names"=w535:string[], "RPM"=w526:dbl[], "TCPCon Out"=w504:refnum<k5>, "tau"=w527:dbl[])  [unwired: 6 in]
                  n171 = call "ReadAltitudeMsg.vi"("TCPCon In"=w504) -> ("Error Out"=w516:errorcluster, "Altitide Estimated"=w446:dbl, "Altitude"=w520:dbl, "TCPCon Out"=w483:refnum<k5>, "Altitude Desired"=w445:dbl, "dvl"=w508:dbl[], "Altitude Proximated"=w511:dbl)  [unwired: 4 in]
                  "Des. Altitude" <- w445
                  "Altitide [m]" <- w446
                  n172 = call "Read Attitude Msg.vi"("TCP  Refnum In"=w483) -> ("MT_DATA"=w493:dbl[], "TCP Refnum Out"=w476:refnum<k5>, "Omega Estimated"=w494:dbl[], "Theta Estimated"=w496:dbl[], "Omega Measured"=w495:dbl[], "Theta Measured"=w497:dbl[])  [unwired: 5 in]
                  n173 = call "Read Ship States.vi"("TCP Refnum In"=w476) -> ("Eta_ship"=w436:dbl[], "TCP Refnum Out"=w439:refnum<k5>)  [unwired: 9 in]
                  n174 = expression code="(x/pi)*180.0" ("radians to degrees")(w564) -> (w563:dbl)
                  "Des Head. [deg]" <- w563
                  n175 = expression code="(x/pi)*180.0" ("radians to degrees")(w579) -> (w578:dbl)
                  "Head. [deg]" <- w578
                  n176 = invoke class="VI" method="Ctrl Val.Set"(reference=w503, error in=w516, "Control Name"="Alt", "Value"=w520) -> (reference out=w522:refnum<vi>, error out=w515:errorcluster)  [unwired: 1 in, 3 out]
                  n177 = Array Subset(array=w573, index=15, length=4) -> (→"ALTITUDE BEAMS":bool[])
                  n178 = property on="Start Button" class="Bool (strict)"() -> ("Value"=w525:bool)  [unwired: 2 in, 2 out]
                  n179 = Write to Text File(file (use dialog)=w478, text=w556) -> (refnum out=w481:refnum<file>)  [unwired: 2 in, 2 out]
                  n180 = Write to Text File(file (use dialog)=w477, text=w553) -> (refnum out=w479:refnum<file>)  [unwired: 2 in, 2 out]
                  n181 = Bundle("Des Depth [m]"=w449, "Depth [m]"=w448) -> (→"DEPTH":cluster{"Des Depth [m]":dbl, "Depth [m]":dbl})  [unwired: 1 in]
                  n182 = Bundle("Des Heading [deg]"=w563, "Heading [deg]"=w578) -> (→"DESIRED (red) / ESTIMATED (blue) HEADING":T6)  [unwired: 1 in]
                  n183 = call "LogThrustStringCreator.vi"("rpm"=w526, "Tau"=w527) -> ("output"=w528:string)
                  n184 = invoke class="VI" method="Ctrl Val.Set"(reference=w503, error in=w531, "Control Name"="Tau", "Value"=w527) -> (reference out=w537:refnum<vi>, error out=w530:errorcluster)  [unwired: 1 in, 3 out]
                  n185 = Bundle("Altitude Desired"=w445, "Altitide Estimated"=w446) -> (→"ALTITUDE":T7)  [unwired: 1 in]
                  n186 = invoke class="VI" method="Ctrl Val.Set"(reference=w522, error in=w515, "Control Name"="Alt_e", "Value"=w446) -> (reference out=w521:refnum<vi>, error out=w514:errorcluster)  [unwired: 1 in, 3 out]
                  n187 = invoke class="VI" method="Ctrl Val.Set"(reference=w589, "Control Name"=w546, "Value"=w545) -> (reference out=w588:refnum<vi>)  [unwired: 2 in, 4 out]
                  n188 = vi-ref "DP Panel.vi"() -> (w583:refnum<vi>)
                  n189 = Set File Position(refnum=w481, from (0:start)=enum16{"start", "end", "current"}."current") -> (refnum out=w557:refnum<file>)  [unwired: 2 in, 1 out]
                  n190 = vi-ref "Tracking Panel.vi"() -> (w435:refnum<vi>)
                  n191 = Set File Position(refnum=w479, from (0:start)=enum16{"start", "end", "current"}."current") -> (refnum out=w552:refnum<file>)  [unwired: 2 in, 1 out]
                  n192 = case shown="True" w525 {
                    tunnel: [w690 w691] -> w524
                    tunnel: w523 -> [w690 w695]
                    tunnel: w528 -> [_ w694]
                    frame False {
                    }
                    frame True {
                      n193 = Write to Text File(file (use dialog)=w695, text=w694) -> (refnum out=w692:refnum<file>)  [unwired: 2 in, 2 out]
                      n194 = Set File Position(refnum=w692, from (0:start)=enum16{"start", "end", "current"}."current") -> (refnum out=w691:refnum<file>)  [unwired: 2 in, 1 out]
                    }
                  }
                  n195 = invoke class="VI" method="Ctrl Val.Set"(reference=w583, "Control Name"=w546, "Value"=w539) -> ()  [unwired: 2 in, 5 out]
                  n196 = invoke class="VI" method="Ctrl Val.Set"(reference=w503, "Control Name"=w546, "Value"=w545) -> (reference out=w570:refnum<vi>, error out=w569:errorcluster)  [unwired: 2 in, 3 out]
                  n197 = invoke class="VI" method="Ctrl Val.Set"(reference=w588, "Control Name"=w540, "Value"=w539) -> (reference out=w551:refnum<vi>)  [unwired: 2 in, 4 out]
                  n198 = invoke class="VI" method="Ctrl Val.Set"(reference=w537, error in=w530, "Control Name"="RPM", "Value"=w526) -> (reference out=w536:refnum<vi>, error out=w529:errorcluster)  [unwired: 1 in, 3 out]
                  n199 = invoke class="VI" method="Ctrl Val.Set"(reference=w521, error in=w514, "Control Name"="Alt_d", "Value"=w445) -> (reference out=w513:refnum<vi>, error out=w507:errorcluster)  [unwired: 1 in, 3 out]
                  n200 = invoke class="VI" method="Ctrl Val.Set"(reference=w570, error in=w569, "Control Name"=w540, "Value"=w539) -> (reference out=w568:refnum<vi>)  [unwired: 1 in, 4 out]
                  n201 = invoke class="VI" method="Ctrl Val.Set"(reference=w568, "Control Name"="Eta_Est", "Value"=w433) -> (reference out=w562:refnum<vi>)  [unwired: 2 in, 4 out]
                  n202 = invoke class="VI" method="Ctrl Val.Set"(reference=w562, "Control Name"="Nu", "Value"=w555) -> (reference out=w585:refnum<vi>)  [unwired: 2 in, 4 out]
                  n203 = invoke class="VI" method="Ctrl Val.Set"(reference=w585, "Control Name"="Nu_e", "Value"=w554) -> (reference out=w561:refnum<vi>)  [unwired: 2 in, 4 out]
                  n204 = invoke class="VI" method="Ctrl Val.Set"(reference=w561, "Control Name"="Nu_d", "Value"=w548) -> (reference out=w559:refnum<vi>)  [unwired: 2 in, 4 out]
                  n205 = invoke class="VI" method="Ctrl Val.Set"(reference=w435, "Control Name"="Eta_Est", "Value"=w433) -> ()  [unwired: 2 in, 5 out]
                  n206 = Index Array(array=w433, index #1=3 ("index"), index #2=4 ("index"), index #3=5 ("index")) -> (element #1=w456:dbl, element #2=w455:dbl, element #3=w451:dbl)
                  n207 = invoke class="VI" method="Ctrl Val.Set"(reference=w536, error in=w529, "Control Name"="Thruster Names", "Value"=w535) -> ()  [unwired: 1 in, 5 out]
                  n208 = invoke class="VI" method="Ctrl Val.Set"(reference=w513, error in=w507, "Control Name"="Alt_a", "Value"=w511) -> (reference out=w510:refnum<vi>, error out=w506:errorcluster)  [unwired: 1 in, 3 out]
                  n209 = invoke class="VI" method="Ctrl Val.Set"(reference=w547, "Control Name"=w546, "Value"=w545) -> (reference out=w544:refnum<vi>, error out=w543:errorcluster)  [unwired: 2 in, 3 out]
                  n210 = expression code="-(x/pi)*180.0" ("radians to degrees")(w456) -> (w454:dbl)
                  n211 = expression code="(x/pi)*180.0" ("radians to degrees")(w455) -> (w453:dbl)
                  n212 = expression code="(x/pi)*180.0" ("radians to degrees")(w451) -> (→"Compass Indicator":dbl)
                  n213 = Bundle("Des Heading [deg]"=w454, "Des Heading [deg]"=w453) -> (→"Attitude Indicator":T8)  [unwired: 1 in]
                  n214 = invoke class="VI" method="Ctrl Val.Set"(reference=w544, error in=w543, "Control Name"=w542, "Value"=w433) -> (reference out=w541:refnum<vi>)  [unwired: 1 in, 4 out]
                  n215 = invoke class="VI" method="Ctrl Val.Set"(reference=w510, error in=w506, "Control Name"="dvl", "Value"=w508) -> (reference out=w502:refnum<vi>)  [unwired: 1 in, 4 out]
                  n216 = invoke class="VI" method="Ctrl Val.Set"(reference=w502, "Control Name"="Theta_M", "Value"=w497) -> (reference out=w501:refnum<vi>, error out=w487:errorcluster)  [unwired: 2 in, 3 out]
                  n217 = invoke class="VI" method="Ctrl Val.Set"(reference=w501, error in=w487, "Control Name"="Theta_E", "Value"=w496) -> (reference out=w500:refnum<vi>, error out=w486:errorcluster)  [unwired: 1 in, 3 out]
                  n218 = invoke class="VI" method="Ctrl Val.Set"(reference=w500, error in=w486, "Control Name"="Omega_M", "Value"=w495) -> (reference out=w499:refnum<vi>, error out=w485:errorcluster)  [unwired: 1 in, 3 out]
                  n219 = invoke class="VI" method="Ctrl Val.Set"(reference=w499, error in=w485, "Control Name"="Omega_E", "Value"=w494) -> (reference out=w498:refnum<vi>, error out=w484:errorcluster)  [unwired: 1 in, 3 out]
                  n220 = invoke class="VI" method="Ctrl Val.Set"(reference=w498, error in=w484, "Control Name"="MT_DATA", "Value"=w493) -> ()  [unwired: 1 in, 5 out]
                  n221 = invoke class="VI" method="Ctrl Val.Set"(reference=w541, "Control Name"=w540, "Value"=w539) -> (reference out=w472:refnum<vi>)  [unwired: 2 in, 4 out]
                  n222 = invoke class="VI" method="Ctrl Val.Set"(reference=w551, "Control Name"=w542, "Value"=w433) -> (reference out=w471:refnum<vi>)  [unwired: 2 in, 4 out]
                  n223 = invoke class="VI" method="Ctrl Val.Set"(reference=w471, "Control Name"=w474, "Value"=w436) -> (reference out=w470:refnum<vi>, error out=w475:errorcluster)  [unwired: 2 in, 3 out]
                  n224 = invoke class="VI" method="Ctrl Val.Set"(reference=w472, error in=w475, "Control Name"=w474, "Value"=w436) -> (reference out=w473:refnum<vi>)  [unwired: 1 in, 4 out]
                  n225 = Bundle(u32 16711680, u32 16711680) -> (w440:cluster{u32, u32})  [unwired: 1 in]
                  n226 = property on="DESIRED (red) / ESTIMATED (blue) HEADING" class="Slide (strict)"("Slider Colors"=w440) -> ()  [unwired: 2 in, 2 out]
                  n227 = property on="DEPTH" class="Slide (strict)"("Slider Colors"=w440) -> ()  [unwired: 2 in, 2 out]
                  n228 = mathscript code="d=sqrt((eta(1)-etaS(1))^2+(eta(2)-etaS(2))^2)\nif d<=25\nwarning=true;\nelse\nwarning=false;\nend"("eta"=w433, "etaS"=w436) -> ("d"=→"Des Head. [deg] 2":cdb, "warning"=→"!":bool)  [unwired: 1 in, 1 out]
                  n229 = property on="ALTITUDE" class="Slide (strict)"("Slider Colors"=w440) -> ()  [unwired: 2 in, 2 out]
                  "SONAR ALT" <- FALSE ("Sonar Alt")
                }
                frame Error {
                  n230 = Unbundle By Name(w721) -> ("code"=w720:i32, "source"=w719:string)  [unwired: 1 out]
                  n231 = property on="Connect Button" class="Bool (strict)"("Val(Sgnl)"=FALSE) -> ()  [unwired: 2 in, 2 out]
                  n232 = call "Build Text4"("Code"=w720, "Source"=w719) -> ("Result"=w718:string)  [unwired: 12 in, 1 out]
                  n233 = call "Display Message to User2"("Message"=w718) -> ("Yes"=w717:bool)  [unwired: 9 in, 1 out]
                }
              }
              n234 = property on="Connect Button" class="Bool (strict)"() -> ("Value"=w421:bool)  [unwired: 2 in, 2 out]
            }
            n235 = vi-ref "Light Panel.vi"() -> (w313:refnum<vi>)
            n236 = vi-ref "Empty Panel.vi"() -> (w312:refnum<vi>)
            n237 = while {
              shift-right: [w754] -> _
              shift-left: w306 -> [w753]
              shift-right: [w752] -> _
              shift-left: w313 -> [w751]
              shift-right: [w743] -> _
              shift-left: w312 -> [w750]
              shift-right: [w745] -> w280
              shift-left: w291 -> [w746]
              tunnel: w277 -> [w744]
              i -> [w748]
              stop <- w747 stop-if-true
              # "Event Handler"
              n238 = event shown="[5] \"Tracking Button\": Value Change" {
                selector: _ -> [_ _ _ _ _ _ _ _ _ _ _ _ _ _ _ _ _ _ _ _ _ _ _ _ _ _ _]
                dyn-events: _ -> [_ _ _ _ _ _ _ _ _ _ _ _ _ _ _ _ _ _ _ _ _ _ _ _ _ _ _]
                timeout: _ -> [_ _ _ _ _ _ _ _ _ _ _ _ _ _ _ _ _ _ _ _ _ _ _ _ _ _ _]
                tunnel: [w758 w764 w779 w796 w808 w818 w829 w846 w857 w868 w877 w887 w893 w899 w903 w908 w913 w924 w952 w958 w969 w976 w989 w1024 w1035 w1059 w1082] -> w743
                tunnel: w750 -> [w758 w764 w779 w796 w807 w820 w830 w846 w857 w868 w877 w887 w893 w899 w903 w908 w913 w924 w952 w958 w969 w976 w989 w1024 w1035 w1059 w1082]
                tunnel: [w757 w766 w780 w797 w810 w822 w834 w845 w856 w867 w875 w888 w894 w900 w904 w909 w914 w925 w953 w959 w968 w977 w990 w1025 w1036 w1060 w1083] -> w752
                tunnel: w751 -> [w757 w766 w780 w797 w810 w822 w834 w842 w853 w864 w874 w888 w894 w900 w904 w909 w914 w925 w953 w959 w968 w977 w990 w1025 w1036 w1060 w1083]
                tunnel: [w756 w765 w781 w798 w809 w821 w833 w844 w855 w866 w878 w889 w895 w901 w905 w910 w915 w926 w954 w960 w967 w978 w991 w1026 w1037 w1061 w1084] -> w754
                tunnel: w753 -> [w756 w765 w781 w798 w809 w821 w833 w844 w855 w866 w878 _ w895 w901 w905 w910 w915 w926 w954 w960 w967 w978 w991 w1026 w1037 w1061 w1084]
                tunnel: [_ _ _ _ _ _ _ _ _ _ _ _ "The connection button. Used to \nconnect to the control system." "The butten used to open\nthe Dynamic Positioning system\npanel" "" "The butten used to open\nthe Joystick\npanel" "The butten used to open\nthe Tracking system panel" _ _ _ _ _ _ _ _ _ _] -> w749
                tunnel: w748 -> [_ _ _ _ _ _ _ _ _ _ _ _ _ _ _ _ _ _ _ _ _ _ _ _ _ _ _]
                tunnel: [_ w759 _ w794 _ _ _ _ _ _ _ _ _ _ _ _ _ _ _ _ _ _ _ _ _ _ _] -> w747
                tunnel: w746 -> [w755 w763 w783 w795 w805 w817 w831 w841 w852 w863 w876 w885 w892 w897 w902 w907 w912 w923 w951 w962 w971 w980 w986 w1018 w1028 w1052 w1076]
                tunnel: [w755 w763 w782 w795 w805 w817 w831 w841 w852 w863 w876 w885 w892 w897 w902 w907 w912 w922 w951 w961 w970 w979 w985 w1017 w1027 w1051 w1075] -> w745
                tunnel: w744 -> [_ _ _ _ _ _ _ _ _ _ _ _ _ _ _ _ _ _ w957 _ _ _ _ _ _ _ _]
                event Timeout {
                  n239 = event-data() -> ()  [unwired: 1 in, 2 out]
                }
                event "Stop Button": Value Change {
                  n240 = event-data() -> ()  [unwired: 1 in, 5 out]
                  n241 = Two Button Dialog(message="Do you want to stop the\ncontrol system?", 1:"No" ("F button name (\"Cancel\")"), 2:"Yes" ("T button name (\"OK\")")) -> (T button?=w759:bool)
                  n242 = property on="Stop Button" class="Bool (strict)"("Value"=w759) -> ()  [unwired: 2 in, 2 out]
                  n243 = Not(x=w759) -> (.not. x?=w767:bool)
                  n244 = property on="Connect Button" class="Bool (strict)"("Value"=w767) -> ()  [unwired: 2 in, 2 out]
                }
                event "SetOrigin": Value Change {
                  w771 = "Output" ("Control Name")
                  n245 = event-data() -> ()  [unwired: 1 in, 5 out]
                  n246 = vi-ref "SetOriginPanel.vi"() -> (w778:refnum<vi>)
                  n247 = invoke class="VI" method="FP.Open"(reference=w778) -> (reference out=w777:refnum<vi>, error out=w776:errorcluster)  [unwired: 4 in, 3 out]
                  n248 = invoke class="VI" method="Run VI"(reference=w777, error in=w776, "Wait until done"=TRUE ("Wait Until Done")) -> (reference out=w773:refnum<vi>, error out=w772:errorcluster)  [unwired: 2 in, 3 out]
                  n249 = invoke class="VI" method="Ctrl Val.Get"(reference=w773, error in=w772, "Control Name"=w771) -> ("Get Control Value Variant"=w774:variant)  [unwired: 1 in, 3 out]
                  n250 = Variant To Data(type=w771, Variant=w774) -> (data=w770:string)  [unwired: 1 in, 1 out]
                  n251 = String Length(string=w770) -> (length=w769:i32)
                  n252 = Greater Than 0?(x=w769) -> (x > 0?=w768:bool)
                  n253 = case shown="True" w768 {
                    tunnel: w783 -> [w784 w787]
                    tunnel: [w784 w786] -> w782
                    tunnel: w770 -> [_ w785]
                    frame False {
                    }
                    frame True {
                      n254 = call "Build Text5"("Origin"=w785) -> ("Result"=w789:string)  [unwired: 13 in, 1 out]
                      n255 = String Length(string=w789) -> (length=w791:i32)
                      n256 = Type Cast(x=w791) -> (*(type *) &x=w790:string)  [unwired: 1 in]
                      n257 = Concatenate Strings(w790, w789) -> (w788:string)
                      n258 = TCP Write(connection ID=w787, data in=w788) -> (connection ID out=w786:refnum<k5>)  [unwired: 2 in, 2 out]
                    }
                  }
                }
                event "Connect Button": Value Change {
                  n259 = event-data() -> ("NewVal"=w793:bool)  [unwired: 1 in, 4 out]
                  n260 = case shown="False" w793 {
                    selector: w793 -> [_ w804]
                    tunnel: [w800 w804] -> w792
                    frame False {
                      n261 = Two Button Dialog(message="Are you sure you want\nto break the connection?", 1:"No" ("F button name (\"Cancel\")"), 2:"Yes" ("T button name (\"OK\")")) -> (T button?=w800:bool)
                      n262 = Not(x=w800) -> (.not. x?=w799:bool)
                      n263 = property on="Connect Button" class="Bool (strict)"("Value"=w799) -> ()  [unwired: 2 in, 2 out]
                    }
                    frame True {
                    }
                  }
                  n264 = Not(x=w792) -> (.not. x?=w794:bool)
                }
                event "DP Button": Value Change {
                  n265 = event-data() -> ("NewVal"=w806:bool)  [unwired: 1 in, 4 out]
                  n266 = case shown="True" w806 {
                    selector: w806 -> [w811 w815]
                    tunnel: [w813 w816] -> w808
                    tunnel: w807 -> [w813 _]
                    frame False {
                      n267 = Not(x=w811) -> (.not. x?=w812:bool)
                      n268 = property on="DP Button" class="Bool (strict)"("Value"=w812) -> ()  [unwired: 2 in, 2 out]
                    }
                    frame True {
                      n269 = Not(x=w815) -> (.not. x?=w814:bool)
                      n270 = vi-ref "DP Panel.vi"() -> (w816:refnum<vi>)
                      n271 = property on="Tracking Button" class="Bool (strict)"("Value"=w814) -> ()  [unwired: 2 in, 2 out]
                      n272 = property on="Joystick Button" class="Bool (strict)"("Value"=w814) -> ()  [unwired: 2 in, 2 out]
                    }
                  }
                }
                event "Tracking Button": Value Change {
                  n273 = event-data() -> ("NewVal"=w819:bool)  [unwired: 1 in, 4 out]
                  n274 = case shown="True" w819 {
                    selector: w819 -> [w823 w828]
                    tunnel: [w825 w826] -> w818
                    tunnel: w820 -> [w825 _]
                    frame False {
                      n275 = Not(x=w823) -> (.not. x?=w824:bool)
                      n276 = property on="Tracking Button" class="Bool (strict)"("Value"=w824) -> ()  [unwired: 2 in, 2 out]
                    }
                    frame True {
                      n277 = Not(x=w828) -> (.not. x?=w827:bool)
                      n278 = vi-ref "Tracking Panel.vi"() -> (w826:refnum<vi>)
                      n279 = property on="Joystick Button" class="Bool (strict)"("Value"=w827) -> ()  [unwired: 2 in, 2 out]
                      n280 = property on="DP Button" class="Bool (strict)"("Value"=w827) -> ()  [unwired: 2 in, 2 out]
                    }
                  }
                }
                event "Joystick Button": Value Change {
                  n281 = event-data() -> ("NewVal"=w832:bool)  [unwired: 1 in, 4 out]
                  n282 = case shown="True" w832 {
                    selector: w832 -> [w836 w839]
                    tunnel: [w837 w840] -> w829
                    tunnel: w830 -> [w837 _]
                    frame False {
                      n283 = Not(x=w836) -> (.not. x?=w835:bool)
                      n284 = property on="Joystick Button" class="Bool (strict)"("Value"=w835) -> ()  [unwired: 2 in, 2 out]
                    }
                    frame True {
                      n285 = Not(x=w839) -> (.not. x?=w838:bool)
                      n286 = vi-ref "HMI Panel.vi"() -> (w840:refnum<vi>)
                      n287 = property on="Tracking Button" class="Bool (strict)"("Value"=w838) -> ()  [unwired: 2 in, 2 out]
                      n288 = property on="DP Button" class="Bool (strict)"("Value"=w838) -> ()  [unwired: 2 in, 2 out]
                    }
                  }
                }
                event "LIGHTS": Value Change {
                  n289 = event-data() -> ()  [unwired: 1 in, 5 out]
                  n290 = case shown="True" "LIGHTS" {
                    selector: "LIGHTS" -> [w848 _]
                    tunnel: [w849 w851] -> w845
                    tunnel: w842 -> [w849 _]
                    frame False {
                      n291 = Not(x=w848) -> (.not. x?=w847:bool)
                      n292 = property on="LIGHTS" class="Bool (strict)"("Value"=w847) -> ()  [unwired: 2 in, 2 out]
                    }
                    frame True {
                      w850 = FALSE
                      n293 = property on="COLLECTION\nUNIT" class="Bool (strict)"("Value"=w850) -> ()  [unwired: 2 in, 2 out]
                      n294 = property on="MANIPULATOR" class="Bool (strict)"("Value"=w850) -> ()  [unwired: 2 in, 2 out]
                      n295 = property on="CAMERAS" class="Bool (strict)"("Value"=w850) -> ()  [unwired: 2 in, 2 out]
                      n296 = vi-ref "Light Panel.vi"() -> (w851:refnum<vi>)
                    }
                  }
                }
                event "MANIPULATOR": Value Change {
                  n297 = event-data() -> ()  [unwired: 1 in, 5 out]
                  n298 = case shown="False" "MANIPULATOR" {
                    selector: "MANIPULATOR" -> [w859 _]
                    tunnel: [w860 w862] -> w856
                    tunnel: w853 -> [w860 _]
                    frame False {
                      n299 = Not(x=w859) -> (.not. x?=w858:bool)
                      n300 = property on="MANIPULATOR" class="Bool (strict)"("Value"=w858) -> ()  [unwired: 2 in, 2 out]
                    }
                    frame True {
                      w861 = FALSE
                      n301 = property on="COLLECTION\nUNIT" class="Bool (strict)"("Value"=w861) -> ()  [unwired: 2 in, 2 out]
                      n302 = property on="LIGHTS" class="Bool (strict)"("Value"=w861) -> ()  [unwired: 2 in, 2 out]
                      n303 = property on="CAMERAS" class="Bool (strict)"("Value"=w861) -> ()  [unwired: 2 in, 2 out]
                      n304 = vi-ref "Manipulator Panel.vi"() -> (w862:refnum<vi>)
                    }
                  }
                }
                event "CAMERAS": Value Change {
                  n305 = event-data() -> ()  [unwired: 1 in, 5 out]
                  n306 = case shown="True" "CAMERAS" {
                    selector: "CAMERAS" -> [w870 _]
                    tunnel: [w871 w873] -> w867
                    tunnel: w864 -> [w871 _]
                    frame False {
                      n307 = Not(x=w870) -> (.not. x?=w869:bool)
                      n308 = property on="CAMERAS" class="Bool (strict)"("Value"=w869) -> ()  [unwired: 2 in, 2 out]
                    }
                    frame True {
                      w872 = FALSE
                      n309 = property on="COLLECTION\nUNIT" class="Bool (strict)"("Value"=w872) -> ()  [unwired: 2 in, 2 out]
                      n310 = property on="MANIPULATOR" class="Bool (strict)"("Value"=w872) -> ()  [unwired: 2 in, 2 out]
                      n311 = property on="LIGHTS" class="Bool (strict)"("Value"=w872) -> ()  [unwired: 2 in, 2 out]
                      n312 = vi-ref "Camera Control.vi"() -> (w873:refnum<vi>)
                    }
                  }
                }
                event "COLLECTION\nUNIT": Value Change {
                  n313 = event-data() -> ()  [unwired: 1 in, 5 out]
                  n314 = case shown="True" "COLLECTION\nUNIT" {
                    selector: "COLLECTION\nUNIT" -> [w882 _]
                    tunnel: [w880 w883] -> w875
                    tunnel: w874 -> [w880 _]
                    frame False {
                      n315 = Not(x=w882) -> (.not. x?=w881:bool)
                      n316 = property on="COLLECTION\nUNIT" class="Bool (strict)"("Value"=w881) -> ()  [unwired: 2 in, 2 out]
                    }
                    frame True {
                      w884 = FALSE
                      n317 = property on="LIGHTS" class="Bool (strict)"("Value"=w884) -> ()  [unwired: 2 in, 2 out]
                      n318 = property on="CAMERAS" class="Bool (strict)"("Value"=w884) -> ()  [unwired: 2 in, 2 out]
                      n319 = property on="MANIPULATOR" class="Bool (strict)"("Value"=w884) -> ()  [unwired: 2 in, 2 out]
                      n320 = vi-ref "Collecting Unit.vi"() -> (w883:refnum<vi>)
                    }
                  }
                }
                event "Vessel Data": Value Change {
                  n321 = event-data() -> ()  [unwired: 1 in, 5 out]
                  n322 = case shown="True" "Vessel Data" {
                    tunnel: [w890 w891] -> w889
                    frame False {
                      n323 = vi-ref "Map Visualization.vi"() -> (w890:refnum<vi>)
                    }
                    frame True {
                      n324 = vi-ref "Vessel Visualization.vi"() -> (w891:refnum<vi>)
                    }
                  }
                }
                event "Connect Button": Mouse Enter {
                  n325 = event-data() -> ()  [unwired: 1 in, 3 out]
                }
                event "DP Button": Mouse Enter {
                  n326 = event-data() -> ()  [unwired: 1 in, 3 out]
                }
                event Mouse Enter {
                  n327 = event-data() -> ()  [unwired: 1 in, 3 out]
                }
                event "Joystick Button": Mouse Enter {
                  n328 = event-data() -> ()  [unwired: 1 in, 3 out]
                }
                event "Tracking Button": Mouse Enter {
                  n329 = event-data() -> ()  [unwired: 1 in, 3 out]
                }
                event "Start Button": Value Change {
                  n330 = event-data() -> ("NewVal"=w918:bool)  [unwired: 1 in, 4 out]
                  n331 = case shown="True" w918 {
                    tunnel: ["0,0,0" w930] -> w921
                    tunnel: [T5."Disabled and Grayed Out" ("Disabled") T5."Enabled" ("Disabled")] -> w917
                    frame False {
                    }
                    frame True {
                      w931 = "Output" ("Control Name")
                      n332 = vi-ref "SetOriginPanel.vi"() -> (w938:refnum<vi>)
                      n333 = invoke class="VI" method="FP.Open"(reference=w938) -> (reference out=w937:refnum<vi>, error out=w936:errorcluster)  [unwired: 4 in, 3 out]
                      n334 = invoke class="VI" method="Run VI"(reference=w937, error in=w936, "Wait until done"=TRUE ("Wait Until Done")) -> (reference out=w934:refnum<vi>, error out=w933:errorcluster)  [unwired: 2 in, 3 out]
                      n335 = invoke class="VI" method="Ctrl Val.Get"(reference=w934, error in=w933, "Control Name"=w931) -> ("Get Control Value Variant"=w932:variant)  [unwired: 1 in, 3 out]
                      n336 = Variant To Data(type=w931, Variant=w932) -> (data=w930:string)  [unwired: 1 in, 1 out]
                    }
                  }
                  n337 = String Length(string=w921) -> (length=w919:i32)
                  n338 = Greater Than 0?(x=w919) -> (x > 0?=w920:bool)
                  n339 = case shown="True" w920 {
                    tunnel: w923 -> [w940 w945]
                    tunnel: w918 -> [_ w944]
                    tunnel: [w940 w943] -> w922
                    tunnel: w921 -> [_ w942]
                    tunnel: w917 -> [_ w941]
                    frame False {
                      n340 = property on="Start Button" class="Bool (strict)"("Value"=FALSE ("Start Button")) -> ()  [unwired: 2 in, 2 out]
                    }
                    frame True {
                      n341 = Boolean To (0,1)(Boolean=w944) -> (0, 1=w950:i16)
                      n342 = call "Build Text7"("Value"=w950, "Origin"=w942) -> ("Result"=w947:string)  [unwired: 12 in, 1 out]
                      n343 = property on="DP Button" class="Bool (strict)"("DisabledEnum"=w941) -> ()  [unwired: 2 in, 2 out]
                      n344 = property on="Joystick Button" class="Bool (strict)"("DisabledEnum"=w941) -> ()  [unwired: 2 in, 2 out]
                      n345 = property on="Tracking Button" class="Bool (strict)"("DisabledEnum"=w941) -> ()  [unwired: 2 in, 2 out]
                      n346 = String Length(string=w947) -> (length=w949:i32)
                      n347 = property on="Reset Plots" class="Bool"("DisabledEnum"=w941) -> ()  [unwired: 2 in, 2 out]
                      n348 = property on="Reset Controller" class="Bool"("DisabledEnum"=w941) -> ()  [unwired: 2 in, 2 out]
                      n349 = property on="Reset Observer" class="Bool"("DisabledEnum"=w941) -> ()  [unwired: 2 in, 2 out]
                      n350 = Type Cast(type=w947, x=w949) -> (*(type *) &x=w948:string)
                      n351 = property on="Reset ROV" class="Bool"("DisabledEnum"=w941) -> ()  [unwired: 2 in, 2 out]
                      n352 = property on="SetOrigin" class="Bool"("DisabledEnum"=w941) -> ()  [unwired: 2 in, 2 out]
                      n353 = Concatenate Strings(w948, w947) -> (w946:string)
                      n354 = TCP Write(connection ID=w945, data in=w946) -> (connection ID out=w943:refnum<k5>)  [unwired: 2 in, 2 out]
                    }
                  }
                }
                event "Reset Plots": Value Change {
                  n355 = event-data() -> ()  [unwired: 1 in, 5 out]
                  n356 = invoke class="VI" method="Ctrl Val.Set"(reference=w957, "Control Name"="Reset Plots", "Value"=TRUE) -> ()  [unwired: 2 in, 5 out]
                }
                event "Reset Observer": Value Change {
                  w964 = "16:"
                  n357 = event-data() -> ()  [unwired: 1 in, 5 out]
                  n358 = String Length(string=w964) -> (length=w966:i32)
                  n359 = Type Cast(x=w966) -> (*(type *) &x=w965:string)  [unwired: 1 in]
                  n360 = Concatenate Strings(w965, w964) -> (w963:string)
                  n361 = TCP Write(connection ID=w962, data in=w963) -> (connection ID out=w961:refnum<k5>)  [unwired: 2 in, 2 out]
                }
                event "Reset Controller": Value Change {
                  w973 = "17:"
                  n362 = event-data() -> ()  [unwired: 1 in, 5 out]
                  n363 = String Length(string=w973) -> (length=w975:i32)
                  n364 = Type Cast(x=w975) -> (*(type *) &x=w974:string)  [unwired: 1 in]
                  n365 = Concatenate Strings(w974, w973) -> (w972:string)
                  n366 = TCP Write(connection ID=w971, data in=w972) -> (connection ID out=w970:refnum<k5>)  [unwired: 2 in, 2 out]
                }
                event "Reset ROV": Value Change {
                  w982 = "16:"
                  n367 = event-data() -> ()  [unwired: 1 in, 5 out]
                  n368 = String Length(string=w982) -> (length=w984:i32)
                  n369 = Type Cast(x=w984) -> (*(type *) &x=w983:string)  [unwired: 1 in]
                  n370 = Concatenate Strings(w983, w982) -> (w981:string)
                  n371 = TCP Write(connection ID=w980, data in=w981) -> (connection ID out=w979:refnum<k5>)  [unwired: 2 in, 2 out]
                }
                event Key Up {
                  n372 = event-data() -> ("ScanCode"=w988:i16, "PlatMods"=w987:T9)  [unwired: 1 in, 5 out]
                  n373 = case shown="38" w988 {
                    tunnel: w987 -> [_ w996 _ _ _ _]
                    tunnel: w986 -> [w992 w994 w1005 w1011 w1013 w1015]
                    tunnel: [w992 w993 w1005 w1011 w1013 w1015] -> w985
                    frame 0, Default {
                    }
                    frame 19 {
                      n374 = Unbundle By Name(w996) -> ("Ctrl"=w995:bool)
                      n375 = case shown="True" w995 {
                        selector: w995 -> [_ w1004]
                        tunnel: w994 -> [w997 w999]
                        tunnel: [w997 w998] -> w993
                        frame False {
                        }
                        frame True {
                          w1002 = "23:"
                          n376 = String Length(string=w1002) -> (length=w1003:i32)
                          n377 = property on="Joystick Button" class="Bool (strict)"("Val(Sgnl)"=w1004) -> ()  [unwired: 2 in, 2 out]
                          n378 = Type Cast(type=w1002, x=w1003) -> (*(type *) &x=w1001:string)
                          n379 = Concatenate Strings(w1001, w1002) -> (w1000:string)
                          n380 = TCP Write(connection ID=w999, data in=w1000) -> (connection ID out=w998:refnum<k5>)  [unwired: 2 in, 2 out]
                        }
                      }
                    }
                    frame 35 {
                      n381 = vi-ref "EasterEgg.vi"() -> (w1009:refnum<vi>)
                      n382 = invoke class="VI" method="FP.Open"(reference=w1009) -> (reference out=w1008:refnum<vi>, error out=w1007:errorcluster)  [unwired: 4 in, 3 out]
                      n383 = invoke class="VI" method="Run VI"(reference=w1008, error in=w1007, "Wait until done"=FALSE ("Wait Until Done")) -> ()  [unwired: 2 in, 5 out]
                    }
                    frame 38 {
                      n384 = property on="LIGHTS" class="Bool (strict)"("Val(Sgnl)"=TRUE) -> ()  [unwired: 2 in, 2 out]
                    }
                    frame 46 {
                      n385 = property on="CAMERAS" class="Bool (strict)"("Val(Sgnl)"=TRUE) -> ()  [unwired: 2 in, 2 out]
                    }
                    frame 50 {
                      n386 = property on="MANIPULATOR" class="Bool (strict)"("Val(Sgnl)"=TRUE) -> ()  [unwired: 2 in, 2 out]
                    }
                  }
                }
                event "Reset Signal \nProcessing": Value Change {
                  n387 = event-data() -> ()  [unwired: 1 in, 5 out]
                  n388 = Boolean To (0,1)(Boolean=TRUE) -> (0, 1=w1023:i16)
                  n389 = call "Build Text13"("Value"=w1023) -> ("Result"=w1019:string)  [unwired: 13 in, 1 out]
                  n390 = String Length(string=w1019) -> (length=w1022:i32)
                  n391 = Type Cast(type=w1019, x=w1022) -> (*(type *) &x=w1020:string)
                  n392 = Concatenate Strings(w1020, w1019) -> (w1021:string)
                  n393 = TCP Write(connection ID=w1018, data in=w1021) -> (connection ID out=w1017:refnum<k5>)  [unwired: 2 in, 2 out]
                }
                event "Altitude Button": Value Change {
                  n394 = event-data() -> ()  [unwired: 1 in, 5 out]
                  n395 = Boolean To (0,1)(Boolean="Altitude Button") -> (0, 1=w1030:i16)
                  n396 = call "Build Text14"("act"=w1030) -> ("Result"=w1029:string)  [unwired: 13 in, 1 out]
                  n397 = case shown="True" "Altitude Button" {
                    selector: "Altitude Button" -> [w1046 _]
                    tunnel: [w1046 w1048] -> w1034
                    tunnel: ["" w1049] -> w1033
                    frame False {
                    }
                    frame True {
                      n398 = vi-ref "AltitudeDialog.vi"() -> (w1050:refnum<vi>)
                      n399 = call "AltitudeDialog.vi"() -> ("Result"=w1049:string, "Cancel Button 2"=w1048:bool)  [unwired: 10 in]
                      n400 = invoke on="Invoke Node" class="VI" method="FP.Open"(reference=w1050) -> ()  [unwired: 4 in, 5 out]
                    }
                  }
                  n401 = Concatenate Strings(w1029, w1033) -> (w1032:string)
                  n402 = case shown="False" w1034 {
                    tunnel: w1032 -> [w1041 _]
                    tunnel: w1028 -> [w1040 w1044]
                    tunnel: [w1038 w1044] -> w1027
                    frame False {
                      n403 = String Length(string=w1041) -> (length=w1043:i32)
                      n404 = Type Cast(x=w1043) -> (*(type *) &x=w1042:string)  [unwired: 1 in]
                      n405 = Concatenate Strings(w1042, w1041) -> (w1039:string)
                      n406 = TCP Write(connection ID=w1040, data in=w1039) -> (connection ID out=w1038:refnum<k5>)  [unwired: 2 in, 2 out]
                    }
                    frame True {
                      n407 = property on="Altitude Button" class="Bool (strict)"("Value"=FALSE) -> ()  [unwired: 2 in, 2 out]
                    }
                  }
                }
                event "Set altitude": Value Change {
                  n408 = event-data() -> ()  [unwired: 1 in, 5 out]
                  n409 = Boolean To (0,1)(Boolean="Set altitude") -> (0, 1=w1054:i16)
                  n410 = call "Build Text15"("act"=w1054) -> ("Result"=w1053:string)  [unwired: 13 in, 1 out]
                  n411 = case shown="True" "Set altitude" {
                    selector: "Set altitude" -> [w1069 _]
                    tunnel: [w1069 w1071] -> w1058
                    tunnel: ["" w1072] -> w1057
                    frame False {
                    }
                    frame True {
                      n412 = vi-ref "AltitudeDialog.vi"() -> (w1073:refnum<vi>)
                      n413 = call "AltitudeDialog.vi"() -> ("Result"=w1072:string, "Cancel Button 2"=w1071:bool)  [unwired: 10 in]
                      n414 = invoke on="Invoke Node" class="VI" method="FP.Open"(reference=w1073) -> ()  [unwired: 4 in, 5 out]
                    }
                  }
                  n415 = Concatenate Strings(w1053, w1057) -> (w1056:string)
                  n416 = case shown="False" w1058 {
                    tunnel: w1056 -> [w1065 _]
                    tunnel: w1052 -> [w1064 w1068]
                    tunnel: [w1062 w1068] -> w1051
                    frame False {
                      n417 = String Length(string=w1065) -> (length=w1067:i32)
                      n418 = Type Cast(x=w1067) -> (*(type *) &x=w1066:string)  [unwired: 1 in]
                      n419 = Concatenate Strings(w1066, w1065) -> (w1063:string)
                      n420 = TCP Write(connection ID=w1064, data in=w1063) -> (connection ID out=w1062:refnum<k5>)  [unwired: 2 in, 2 out]
                    }
                    frame True {
                    }
                  }
                }
                event "Start New LogFile": Value Change {
                  n421 = event-data() -> ()  [unwired: 1 in, 5 out]
                  n422 = Boolean To (0,1)(Boolean="Start New LogFile") -> (0, 1=w1081:i16)
                  n423 = call "Build Text8"("Value"=w1081) -> ("Result"=w1077:string)  [unwired: 13 in, 1 out]
                  n424 = String Length(string=w1077) -> (length=w1080:i32)
                  n425 = Type Cast(type=w1077, x=w1080) -> (*(type *) &x=w1078:string)
                  n426 = Concatenate Strings(w1078, w1077) -> (w1079:string)
                  n427 = TCP Write(connection ID=w1076, data in=w1079) -> (connection ID out=w1075:refnum<k5>)  [unwired: 2 in, 2 out]
                }
              }
              "Help Field" <- w749
              n428 = invoke on="Mission Control" class="SubPanel" method="Insert VI"("VI Ref"=w743) -> ()  [unwired: 3 in, 4 out]
              n429 = invoke on="Control Panel" class="SubPanel" method="Insert VI"("VI Ref"=w752) -> ()  [unwired: 3 in, 4 out]
              n430 = invoke on="Map/Vessel Data" class="SubPanel" method="Insert VI"("VI Ref"=w754) -> ()  [unwired: 3 in, 4 out]
            }
            n431 = while {
              tunnel: w298 -> [w320]
              tunnel: w291 -> [w315]
              stop <- w316 continue-if-true
              # "Menu Bar Loop"
              n432 = Get Menu Selection(0:w320) -> (4:w319:bool, 5:w317:refnum<k9>, 6:w318:string)  [unwired: 3 in, 2 out]
              n433 = case shown="False" w319 {
                tunnel: w318 -> [w325 _]
                tunnel: w317 -> [w324 _]
                tunnel: w315 -> [w321 _]
                frame False {
                  n434 = Get Menu Item Info(7:w325, 11:w324) -> (2:w323:string, 3:w322:refnum<k9>)  [unwired: 1 in, 5 out]
                  n435 = case shown="\"Tuning\"" w323 {
                    tunnel: w322 -> [_ _ _ _ _ _ _ _ _ _ _ _ _ _ _]
                    tunnel: w321 -> [w327 _ _ _ _ _ _ _ w349 w355 _ _ _ w382 w385]
                    frame "Extra Buttons" {
                      n436 = vi-ref "Extra Buttons.vi"() -> (w331:refnum<vi>)
                      n437 = invoke class="VI" method="Ctrl Val.Set"(reference=w331, "Control Name"="TCPExtRef", "Value"=w327) -> (reference out=w332:refnum<vi>)  [unwired: 2 in, 4 out]
                      n438 = invoke class="VI" method="FP.Open"(reference=w332) -> (reference out=w330:refnum<vi>, error out=w326:errorcluster)  [unwired: 4 in, 3 out]
                      n439 = invoke class="VI" method="Run VI"(reference=w330, error in=w326, "Wait until done"=FALSE ("Wait Until Done")) -> ()  [unwired: 2 in, 5 out]
                    }
                    frame "~", Default {
                    }
                    frame "Exit" {
                      n440 = property on="Stop Button" class="Bool (strict)"("Val(Sgnl)"=TRUE) -> ()  [unwired: 2 in, 2 out]
                    }
                    frame "About" {
                      n441 = vi-ref "About.vi"() -> (w337:refnum<vi>)
                      n442 = invoke class="VI" method="FP.Open"(reference=w337) -> (reference out=w336:refnum<vi>, error out=w335:errorcluster)  [unwired: 4 in, 3 out]
                      n443 = invoke class="VI" method="Run VI"(reference=w336, error in=w335, "Wait until done"=FALSE ("Wait Until Done")) -> ()  [unwired: 2 in, 5 out]
                    }
                    frame "User Guide" {
                      n444 = vi-ref "Help Center.vi"() -> (w341:refnum<vi>)
                      n445 = invoke class="VI" method="FP.Open"(reference=w341) -> (reference out=w340:refnum<vi>, error out=w339:errorcluster)  [unwired: 4 in, 3 out]
                      n446 = invoke class="VI" method="Run VI"(reference=w340, error in=w339, "Wait until done"=FALSE ("Wait Until Done")) -> ()  [unwired: 2 in, 5 out]
                    }
                    frame "Joystick" {
                      n447 = property on="Joystick Button" class="Bool (strict)"() -> ("Value"=w343:bool)  [unwired: 2 in, 2 out]
                      n448 = Not(x=w343) -> (.not. x?=w342:bool)
                      n449 = property on="Joystick Button" class="Bool (strict)"("Val(Sgnl)"=w342) -> ()  [unwired: 2 in, 2 out]
                    }
                    frame "DP Operation" {
                      n450 = property on="DP Button" class="Bool (strict)"() -> ("Value"=w345:bool)  [unwired: 2 in, 2 out]
                      n451 = Not(x=w345) -> (.not. x?=w344:bool)
                      n452 = property on="DP Button" class="Bool (strict)"("Val(Sgnl)"=w344) -> ()  [unwired: 2 in, 2 out]
                    }
                    frame "Tracking" {
                      n453 = property on="Tracking Button" class="Bool (strict)"() -> ("Value"=w347:bool)  [unwired: 2 in, 2 out]
                      n454 = Not(x=w347) -> (.not. x?=w346:bool)
                      n455 = property on="Tracking Button" class="Bool (strict)"("Val(Sgnl)"=w346) -> ()  [unwired: 2 in, 2 out]
                    }
                    frame "Options" {
                      n456 = vi-ref "Options Panel.vi"() -> (w351:refnum<vi>)
                      n457 = invoke class="VI" method="Ctrl Val.Set"(reference=w351, "Control Name"="TCPOptRef", "Value"=w349) -> (reference out=w350:refnum<vi>)  [unwired: 2 in, 4 out]
                      n458 = invoke class="VI" method="FP.Open"(reference=w350) -> (reference out=w354:refnum<vi>, error out=w353:errorcluster)  [unwired: 4 in, 3 out]
                      n459 = invoke class="VI" method="Run VI"(reference=w354, error in=w353, "Wait until done"=FALSE ("Wait Until Done")) -> ()  [unwired: 2 in, 5 out]
                    }
                    frame "Tuning" {
                      n460 = vi-ref "TuningPanel.vi"() -> (w358:refnum<vi>)
                      n461 = invoke class="VI" method="Ctrl Val.Set"(reference=w358, "Control Name"="TCPConRef", "Value"=w355) -> (reference out=w357:refnum<vi>)  [unwired: 2 in, 4 out]
                      n462 = invoke class="VI" method="FP.Open"(reference=w357) -> (reference out=w361:refnum<vi>, error out=w360:errorcluster)  [unwired: 4 in, 3 out]
                      n463 = invoke class="VI" method="Run VI"(reference=w361, error in=w360, "Wait until done"=FALSE ("Wait Until Done")) -> ()  [unwired: 2 in, 5 out]
                    }
                    frame "Connect" {
                      # "f5 stop button disabled by Fredrik"
                      n464 = case shown="True" FALSE {
                        frame False {
                        }
                        frame True {
                          n465 = property on="Connect Button" class="Bool (strict)"() -> ("Value"=w364:bool)  [unwired: 2 in, 2 out]
                          n466 = Not(x=w364) -> (.not. x?=w363:bool)
                          n467 = property on="Connect Button" class="Bool (strict)"("Val(Sgnl)"=w363) -> ()  [unwired: 2 in, 2 out]
                        }
                      }
                    }
                    frame "Advanced View" {
                      n468 = vi-ref "GraphView.vi"() -> (w367:refnum<vi>)
                      n469 = property on="AdvViewAct" class="Bool (strict)"() -> ("Value"=w366:bool)  [unwired: 2 in, 2 out]
                      n470 = case shown="True" w366 {
                        tunnel: w367 -> [w368 w369]
                        frame False {
                          n471 = invoke class="VI" method="FP.Open"(reference=w368) -> ()  [unwired: 4 in, 5 out]
                        }
                        frame True {
                          n472 = invoke class="VI" method="FP.Close"(reference=w369) -> ()  [unwired: 2 in, 3 out]
                        }
                      }
                      n473 = Not(x=w366) -> (.not. x?=→"AdvViewAct":bool)
                    }
                    frame "Map Window" {
                      n474 = property on="MapViewAct" class="Bool (strict)"() -> ("Value"=w370:bool)  [unwired: 2 in, 2 out]
                      n475 = vi-ref "MapOwnWindow.vi"() -> (w372:refnum<vi>)
                      n476 = case shown="False" w370 {
                        tunnel: w372 -> [w373 w374]
                        frame False {
                          n477 = invoke class="VI" method="FP.Open"(reference=w373) -> ()  [unwired: 4 in, 5 out]
                        }
                        frame True {
                          n478 = invoke class="VI" method="FP.Close"(reference=w374) -> ()  [unwired: 2 in, 3 out]
                        }
                      }
                      n479 = Not(x=w370) -> (.not. x?=→"MapViewAct":bool)
                    }
                    frame "Use Observer" {
                      n480 = property on="Using Observer" class="Bool (strict)"() -> ("Value"=w381:bool)  [unwired: 2 in, 2 out]
                      n481 = Not(x=w381) -> (.not. x?=w380:bool)
                      "Using Observer" <- w380
                      n482 = Boolean To (0,1)(Boolean=w380) -> (0, 1=w379:i16)
                      n483 = call "Build Text6"("Boolean"=w379) -> ("Result"=w376:string)  [unwired: 13 in, 1 out]
                      n484 = String Length(string=w376) -> (length=w378:i32)
                      n485 = Type Cast(x=w378) -> (*(type *) &x=w377:string)  [unwired: 1 in]
                      n486 = Concatenate Strings(w377, w376) -> (w375:string)
                      n487 = TCP Write(connection ID=w382, data in=w375) -> ()  [unwired: 2 in, 3 out]
                    }
                    frame "Use Auto Parameters on Reference Model" {
                      n488 = property on="Auto Par. on Reference Model" class="Bool (strict)"() -> ("Value"=w383:bool)  [unwired: 2 in, 2 out]
                      n489 = Not(x=w383) -> (.not. x?=w384:bool)
                      "Auto Par. on Reference Model" <- w384
                      n490 = Boolean To (0,1)(Boolean=w384) -> (0, 1=w390:i16)
                      n491 = call "Build Text10"("Boolean"=w390) -> ("Result"=w387:string)  [unwired: 13 in, 1 out]
                      n492 = String Length(string=w387) -> (length=w389:i32)
                      n493 = Type Cast(x=w389) -> (*(type *) &x=w388:string)  [unwired: 1 in]
                      n494 = Concatenate Strings(w388, w387) -> (w386:string)
                      n495 = TCP Write(connection ID=w385, data in=w386) -> ()  [unwired: 2 in, 3 out]
                    }
                  }
                }
                frame True {
                }
              }
              n496 = property on="Connect Button" class="Bool (strict)"() -> ("Value"=w316:bool)  [unwired: 2 in, 2 out]
            }
            n497 = while {
              shift-right: [w395] -> _
              shift-left: w300 -> [w396]
              stop <- w394 continue-if-true
              # "Error Message Loop"
              n498 = Dequeue Element(queue=w396, timeout in ms (-1)=100) -> (queue out=w395:refnum<queue>, element=w393:cluster{string, string}, timed out?=w391:bool)  [unwired: 1 in, 1 out]
              n499 = case shown="False" w391 {
                tunnel: w393 -> [w400 _]
                frame False {
                  n500 = Unbundle(w400) -> (w399:string, w398:string)
                  n501 = call "Build Text2"("Time"=w398, "Msg"=w399) -> ("Result"=w397:string)  [unwired: 12 in, 1 out]
                  n502 = One Button Dialog(message=w397) -> ()  [unwired: 1 in, 1 out]
                }
                frame True {
                }
              }
              n503 = property on="Connect Button" class="Bool (strict)"() -> ("Value"=w394:bool)  [unwired: 2 in, 2 out]
            }
          }
          frame Error {
            n504 = Unbundle By Name(w1092) -> ("code"=w1095:i32, "source"=w1094:string)  [unwired: 1 out]
            n505 = call "Build Text3"("Code"=w1095, "Source"=w1094) -> ("Result"=w1091:string)  [unwired: 12 in, 1 out]
            n506 = property on="Connect Button" class="Bool (strict)"("Value"=FALSE ("Connect Button")) -> ()  [unwired: 2 in, 2 out]
            n507 = call "Display Message to User3"("Message"=w1091) -> ("Yes"=w1090:bool)  [unwired: 9 in, 1 out]
          }
        }
      }
      frame #2 {
        # "Finalizing program"
        n508 = case shown="No Error" w1106 {
          tunnel: w1109 -> [w1120 w1124]
          tunnel: w1108 -> [w1116 w1123]
          tunnel: [w1111 w1124] -> w1103
          tunnel: [w1110 w1123] -> w1102
          frame No Error {
            w1112 = -1 ("timeout ms (25000)")
            w1117 = "1:"
            n509 = String Length(string=w1117) -> (length=w1119:i32)
            n510 = vi-ref "Stop VIs.vi"() -> (w1113:refnum<vi>)
            n511 = Type Cast(x=w1119) -> (*(type *) &x=w1118:string)  [unwired: 1 in]
            n512 = invoke class="VI" method="Run VI"(reference=w1113, "Wait until done"=TRUE ("Wait Until Done")) -> ()  [unwired: 3 in, 5 out]
            n513 = Concatenate Strings(w1118, w1117) -> (w1115:string)
            n514 = TCP Write(connection ID=w1116, data in=w1115, 9:w1112) -> (connection ID out=w1110:refnum<k5>)  [unwired: 1 in, 2 out]
            n515 = TCP Write(connection ID=w1120, data in=w1115, 9:w1112) -> (connection ID out=w1111:refnum<k5>)  [unwired: 1 in, 2 out]
          }
          frame Error {
            n516 = vi-ref "Stop VIs.vi"() -> (w1121:refnum<vi>)
            n517 = invoke class="VI" method="Run VI"(reference=w1121, "Wait until done"=TRUE ("Wait Until Done")) -> ()  [unwired: 3 in, 5 out]
            n518 = property on="Stop Button" class="Bool (strict)"("Value"=TRUE ("Stop Button")) -> ()  [unwired: 2 in, 2 out]
          }
        }
        n519 = Close File(refnum=w1099) -> ()  [unwired: 1 in, 2 out]
        n520 = Release Queue(queue=w1107) -> ()  [unwired: 2 in, 3 out]
        n521 = Close File(refnum=w1104) -> ()  [unwired: 1 in, 2 out]
        n522 = Close File(refnum=w1101) -> ()  [unwired: 1 in, 2 out]
        n523 = Close File(refnum=w1100) -> ()  [unwired: 1 in, 2 out]
      }
      frame #3 {
        n524 = property on="Stop Button" class="Bool (strict)"() -> ("Value"=w1129:bool)  [unwired: 2 in, 2 out]
        n525 = TCP Close Connection(connection ID=w1127) -> ()  [unwired: 2 in, 2 out]
        n526 = TCP Close Connection(connection ID=w1126) -> ()  [unwired: 2 in, 2 out]
        n527 = case shown="True" w1129 {
          tunnel: w1128 -> [_ w1131]
          frame False {
          }
          frame True {
            n528 = flat-sequence {
              tunnel: w1131 -> [w1133]
              tunnel: [w1132] -> w1130
              tunnel: w1130 -> [_]
              frame #0 {
                n529 = case shown="True" w1133 {
                  selector: w1133 -> [w1134 _]
                  tunnel: [w1134 w1135] -> w1132
                  frame False {
                  }
                  frame True {
                    w1135 = FALSE ("Wait Until Done")
                    n530 = vi-ref "Restart Procedure.vi"() -> (w1136:refnum<vi>)
                    n531 = invoke class="VI" method="Run VI"(reference=w1136, "Wait until done"=w1135) -> ()  [unwired: 3 in, 5 out]
                  }
                }
              }
              frame #1 {
                n532 = control-ref of="This VI"() -> (w1137:refnum<vi>)
                n533 = invoke class="VI" method="Abort VI"(reference=w1137) -> ()  [unwired: 2 in, 3 out]
              }
            }
          }
        }
      }
    }
  }
